vi "Doktorarbeit_Cornelius.vi"(0 "Heizer":refnum<visa-resource-name>="COM1", 1 "Setpoint\n START":bool, 2 "Write to File":bool, 3 "SP 1 shall be (°C)":dbl=20.0 min=0.0 max=999.0, 4 "Intervall (s)":u32=1 max=600, 5 "Write/\nRead":bool=TRUE, 6 "Delay (ms)":u32=500 min=100 max=600000, 7 "Auto Tune":bool, 9 "Standby":bool, 11 "Reset\nSTOPP":bool, 12 "Read Temperature":bool=TRUE, 13 "Get Values":bool, 15 "File Path":path) -> (8 "Temperature (°C)":dbl format="%#.3f", 14 "SP 1 is (°C)":dbl)   [LabVIEW 2010]
doc: "1. Verwendung\n\nDas Programm dient der Steuerung und Abfrage des Thermocontrollers I3252 und dem Auslesen von zwei VC 840 Messgeräten und einem Druckmessgerät Pfeiffer Single Gauge. \nDie Messgeräte werden Standardmäßig ausgelesen und erst nach Betätigung des Schalters \"Write to File\" in einer Textdatei abgespeichert. Das Eingabefeld \"Intervall\" legt den Abstand der Messpunkte fest.\nDer Setpoint für den Thermocontroller wird erst nach Betätigung des Tasters \"Setpoint START\" übernommen und angesteuert. Er wird ind den EEPROM des Gerätes geschrieben. Die Regelung kann mit Hilfe des Schalters \"Standby\" unterbrochen werden. Durch den Taster \"Reset STOPP\" kann der Setpoint aus dem EEPROM gelöscht werden.\nDie Eingabeflächen \"Constant\" und \"Thickness\" dienen der Berechnung des spezifischen Widerstands.\nDie Eingabeflächen \"User\" und \"Sample\" werden in den Header der Textdatei übernommen.\nDer Indikator \"File Path\" zeigt den aktuellen Speicherort der Textdatei an. Dieser wird nach ausschalten des Schalters \"Write to File\" gelöscht. Bei erneuten Schreiben muss ein neuer Speicherort gewählt werden. Bei Wahl desselben Speicherorts werden sämtliche bereits gespeicherte Daten gelöscht.\n\n\n2. Erläuterungen zum Blockdiagramm\n2.1 äußere Sequenz\nDie äußerte Sequenz besteht aus fünf Frames. Der erste dient der Initialisierung der Ports. Der zweite dient als Verzögerung um dem Programm genug Zeit zu geben die Ports zu öffnen. Jedoch senden die beiden VC 840 bereits Informationen an den Computer die in einem Puffer zwischengespeichert werden. Im dritten Frame wird dieser Puffer geleert. Somit kommt es zu keinem Framing Error. Desweiteren wird in diesem Frame die Startzeit der Messungen genommen. Im vierten Frame wird die eigentliche Messung und Verarbeitung der Daten durchgeführt. Die while-Schleife wird nur durch Auftreten eines Fehlers oder durch Betätigung des Stopbuttons auf dem Front Panel in der oberen linken Ecke unterbrochen. Im fünften und letzten Frame werden die Ports wieder geschlossen und beim Auftreten eines Fehlers wird das Programm automatisch gestoppt. Falls kein Fehler auftritt wird die Sequenz von vorne abgearbeitet.\n\n2.2 while-Schleife und innere Sequenz\n2.2.1 \"Event Structure\"\n2.2.1.1 Allgemein\nDer erste Frame beinhaltet ein \"Event Structure\". Dieser reagiert auf insgesamt elf verschiedene Ereignisse. Falls keines dieser Ereignisse auftreten sollte, warte die Struktur eine Millisekunde bevor die \"Event Structure\" verlassen wird. Die übrigen Ereignisse treten ein, wenn der entsprechende Kontroller eine Werteänderung erfährt.\n\n2.2.1.2 Event: Setpoint\nDieser Case besteht von außen nach innen aus einer Stacked Sequence, einer for-Loop und einer Flat Sequence die wiederum zwei \"Case Structures\" enthält. Als erstes wird bei dem Schalter \"Setpoint START\" der Blinkmodus aktiviert und bei dem Schalter \"Read Temperature\" deaktiviert. Danach folgt das eigentliche setzen des Temperatursollwerts. In der ersten Iteration wird dem Controller I3252 ein Schreibbefehl gesendet. Theoretisch kann der Setpoint in den RAM oder in den EEPROM geschrieben werden. Diese Auswahl erfolgt mit Hilfe des Schalters \"RAM\". Da das Schreiben in den RAM -Speicher aber aus diversen Gründen nicht erwünscht ist, wurde es nicht implementiert. Eine nachträgliche Implementierung ist aber leicht möglich, in dem die untere String-Konstante \"*P012\" durch \"*W012\" ersetzt wird. An diesem Befehl wird eine fünfstellige Hexadezimalzahl angehängt, die den Sollwert wiedergibt. Der Sollwert wird vorher mit zehn multipliziert, da das Komma standardmäßig nach der ersten Ziffer festgesetzt wurde (Bsp.: 800 wird gesendet um 80 einzustellen). Dieser Befehlsstrang wird an das Gerät mittels des SubVIs \"Comm_Interface\", auf welches später noch näher eingegangen wird, weitergegeben. Der durch das Gerät zurückgegebene String wird nicht verarbeitet.\nDie zweite Iteration dient dem Auslesen des eingestellten Sollwertes. Wahlweise kann der RAM- oder der EEPROM-Speicher ausgelesen werden. Die eigentliche Verarbeitung des Ausgabestrings erfolgt durch das SubVI \"Edit Setpoint\".\nDie Implementierung zur Einstellung des zweiten Setpoints erfolgt durch kopieren der ersten beiden Fälle und ersetzen der \"1\" im Befehf durch eine \"2\" (Bsp.: \"*P012\" zu \"*P022\"). Es darf aber nicht vergessen werden, dass dann ebenfalls die Anzahl der Iterationen angepasst werden muss.\nAls letztes wird der Blinkmodus des Schalters \"Setpoint START\" wieder deaktiviert.\n\n2.2.1.3 Event: Standby\nDieses Ereignis aktiviert bzw. deaktiviert als erstes den Blinckmodus des entsprechenden Schalters und sendet danach den Befehl zum aktivieren (\"*D03\") oder zum deaktivieren (\"*E03\") des Standbymodus an den Thermocontroller.\n\n2.2.1.4 Event: Set Command \nDer in das Feld \"Command shall be\" eingegebene Befehl wird an den Thermocontroller übermittlet. Die korrekte Form des Befehls ist im \"Communication Manuel\" nachzuschlagen. Das \"*\"-Zeichen wurde allerdings schon implementiert und muss somit nicht mit eingegeben werden.\n\n2.2.1.5 Event: Reset\nIn der ersten Iteration wird der Reset-Befehl an den Thermocontroller gesendet. In Folge wird der gesamte EEPROM-Speicher gelöscht. Deshalb wird in der zweiten Iteration der Setpoint aktualisiert. Dieser Befehl hat keinen Einfluss auf den RAM-Speicher. Die anschließende Wartezeit ist auf vier Sekunden festgesetzt und wurde empirisch ermittelt. Diese Zeit benötigt das Gerät um den Reset durchzuführen und für die Kommunikation wieder zur Verfügung zu stehen.\n\n2.2.1.6 Event: Auto Tune\nEs ist festgeschrieben, dass der Setpoint für die \"Auto Tune\"-Funktion wenigstens 20°C über der aktuellen Temperatur liegt. Deshalb wird zunächst der aktuelle Temperaturwert ausgelesen. Im zweiten Schritt werden zu diesem Wert zwanzig addiert und der Setpoint wird in den RAM-Speicher geschrieben. Das Schreiben in diesen Speicher ist nötig, da die \"Auto Tune\"-Funktion\" erst nach einem Reset startet. Im dritten Schritt wird der eigentliche Befehl für den \"Auto Tune\" gesendet (siehe dazu \"Communication Manuel\" S.27). Als vierte und letzte Iteration der for-Schleife folgt der bereits erwähnte Reset-Befehl. Der Temperatursollwert, der im RAM-Speicher eingetragen ist, muss zum Schluss wieder auf 0°C gesetzt werden. Die Zeit für die Ausführung des \"Auto Tune\"-Befehls wurde empirisch ermittelt und 45 s festgesetzt.\n\n2.2.1.7 Event: Write LOW/HI\nDieses Ereignis setzt die am Analogausgang anliegende Spannung fest. Normalerweise beträgt dieser Spannungswert 0-10 V. Das angeschlossene Netzteil verträgt aber maximal nur 2,3 V. Aus diesem Grund wird der \"%HIGH\" auf 23 gesetzt. Somit beträgt die maximal anliegende Spannung nur noch 23% von der maximal möglichen, d.h 2,3V. Ein niedrigerer Wert ist jederzeit möglich, genauso wie ein höherer für den Parameter \"%LOW\". Diese werden zunächst nacheinander in den RAM-Speicher geschrieben und anschließend wieder ausgelesen.\n\n2.2.1.8 Event: Set PID\nDie Werte für den PID-Regler können sowohl mit Hilfe der \"Auto Tune\"-Funktion, als auch manuell eingestellt werden. Es wird wiederum zwischen dem Schreiben in den RAM- und dem EEPROM-Speicher unterschieden. Zunächst werden die Werte für \"P\", \"I\" und \"D\", in dieser Reihenfolge, gesetzt und danach die aktuellen Werte ausgelesen.\n\n2.2.1.9 Event: Get Values\nDieses Ereignis hat zur Folge, dass die Werte für \"P\", \"I\", \"D\", \"%LOW\", \"%HIGH\" und des Setpoints wahlweise aus dem RAM- oder EEPROM-Speicher gelesen werden. Die aktuellen Werte werden nicht nur in die entsprechenden Anzeigefelder übernommen, sondern auch in die entsprechenden Eingabefelder, mit Ausnahme des Temperatursollwerts. \n\n2.2.1.10 Event: RAM\nPrinzipiell kann zwischen dem Schreiben in den RAM- oder EEPROM-Speicher des Thermocontrollers gewählt werden. Die entsprechende Schalterposition auf dem Frontpanel zeigt den aktuell verwendeten Speicher an. Die Anzeigewerte werden bei jedem Umschalten aktualisiert und sind im entsprechenden Speicher eingetragen. Die Implementierung ist identisch mit der des Ereignisses \"Get Values\". Es gilt zu beachten, dass die Werte für \"%LOW\" und \"%HIGH\" nur in den RAM-Speicher geschrieben werden können und somit auch nur aus diesem ausgelesen werden können.\n\n2.2.1.11 Event: Set Gauge to Zero\nMit Hilfe der SubVIs \"Get Pressure\" und \"Offset Display\" werden die Werte für den alten und den neuen Offset und der durch den zweiten Drucksensor ermittelt Druck ermittelt. \n\n2.2.1.12 Event: Write to File\nSollte der Schalter \"Write to File\" aktiviert werden, d.h. Schalterposition oben, so wird zunächst durch das SubVI \"Header\" ein Header für die unter \"File Path\" definierte Datei angelegt. Alle Werte, die bereits in der entsprechenden Datei stehen, werden dabei gelöscht.\n\n2.2.2 \"Timed Structures\"\nIm dritten Frame der inneren Sequenz werden die Werte für Zeitpunkt, Temperatur, Spannung, Strom und Druck ermittelt. Damit die Werte zum gleichen Zeitpunkt aufgenommen werden, werden \"Timed Sequences\" eingesetzt. Mit dem entsprechenden Schalter auf dem Front Panel unter dem Tab \"Settings\" kann gewählt werden, ob das entsprechende Gerät ausgelesen werden soll oder nicht. Die einzelnen Sequenzen werden parallel abgearbeitet, womit die Prozesszeit von diesem Frame durch der zeitintensivsten Sequenz abhängt. Dies ist in aller Regel das Auslesen der Temperatur, da ein \"Delay\" von 500 ms oder größer benötigt wird, um den Controller ordentlich ansprechen zu können.\nDie Systemzeit wird durch das SubVI \"System Time in Seconds\" in Sekunden umgerechnet und der in dem Parameter \"Starttime\" gespeicherte Wert wird abgezogen. Somit werden die Sekunden seit dem Start des Programms gezählt.\n\n2.2.3 restlichen Frames\nIm zweiten Frame wird das Intervall zwischen den einzelnen Messwerten festgelegt. Dabei wird der Wert des Parameters \"Delay\" abgezogen. Dieser Wert beträgt im Normalfall 500 ms und ist somit nicht vernachlääsigbar.\nDer Vierte Frame beinhaltet die Umrechnung des Temperatur-Strings in einen Temperaturwert durch das SubVI \"Edit Tmperature\", die Berechnung des spezifischen Widerstands durch das SubVI \"Resistivity Calculation\" und die Überprüfung des Druckwerts. Auch werden die neu gewonnen Werte in das entsprechende Shift-Register übernommen. Falls der Druckwert einen in dem Parameter \"Pressure Limit (mbar)\" festgelegten Grenzwert überschreiten sollte, wird der Thermocontroller automatisch in den Standby-Modus versetzt. Des Weiteren wird der Schalter \"Standby\" solange gesperrt, wie der Druck oberhalb des Grenzwertes liegt. Wenn der Druck wieder unter den Grenzwert gesunken ist, wird der Standby-Befehl nicht automatisch aufgehoben, sondern muss vom Benutzer durch Betätigung des entsprechenden Schalters gegeben werden.\nIm fünften Frame werden die Diagramme erstellt. Dabei wird jedes Mal von neuem das gesamte Shift-Register als Graph dargestellt. Weiterhin werden die Messwerte in ein 1D-Array geschrieben.\nDer sechste und letzte Frame beinhaltet den eigentlich Schreibvorgang der Messwerte in eine Textdatei und die Überprüfung ob ein Fehler vorliegt.\n\n2.3 SubVIs\n2.3.1 Allgemein\nDie SubVIs für die Messgeräte VC840 und das Druckmessgerät wurden aus anderen Quellen übernommen. \n\n2.3.2 \"Header\"\nIn den Header wird zunächst das aktuelle Datum und die aktuelle Zeit übernommen. Die ausgewählte Datei wird dabei überschrieben. Danach wird der Name des Benutzers und der Probe übernommen. Zum Schluss werden die Einheiten in einer Reihe, durch einen Tabulator getrennt, in den Header geschrieben.\n\n2.3.3 \"I3252 Comm Interface\"\nDieses VI stellt die Kommunikation mit dem Thermocontroller her und gibt den Ausgabe-String zurück.\n\n2.3.4 \"I3252 Edit Setpoint\"\nIm Ausgabe-String vom Thermocontroller ist an der vierten Stelle die Stelle des Dezimalpunktes verschlüsselt. Dieses Hexadezimalzahl wird herausgefiltert und an ein \"ENUM Controller\" übergeben. Dieser weist der Hexadezimalzahl eine Nummer zu, mit welcher ein Wert aus einem Array entnommen wird. Dieser Wert dient als Quotient. Der tatsächliche Wert kann somit errechnet werden.\n\n2.3.5 \"I3252 Edit Temperature\"\nDer Temperatur-String, der vom Thermocontroller zurückgegeben wird, wird in eine Dezimalzahl umgewandelt. Manchmal kommt es aus zu Dropouts, die durch dieses Programm herausgefiltert werden. Der letzte Wert wird dabei in einer \"Feedback Node\" gehalten unter der Annahme, dass sich der Temperaturwert nicht sprunghaft ändert.\n\n2.3.6 \"Resistivity Calculation\"\nDer spezifische Widerstand wird nach folgender Formel ausgerechnet. Dabei entspricht t der Dicke der Probe und C ist eine Konstante.\nrho=C*pi*t*U/(ln( 2)*I)\n\n2.3.7 \"System Time in Seconds\"\nZunächst wird die aktuelle Systemzeit ausgelesen. Danach wird diese in Stunden, Minuten und Sekunden aufgeteilt, alles in Sekunden umgerechnet und letztendlich addiert."
uses:
  <vilib>/Platform/TimedLoop/XDataNode/XDataNode.xnode
  <vilib>/Platform/TimedLoop/XDataNode/timing_clust.ctl
  <vilib>/Platform/TimedLoop/XDataNode/nitl_modes.ctl
  <vilib>/Platform/TimedLoop/XDataNode/wakeup.ctl
  <vilib>/Instr/_visa.llb/VISA Configure Serial Port (Instr).vi
  <vilib>/Platform/TimedLoop/scheduler/LVUserAPI/_suppVIs/Create_1kHz_TSource.vi
  <vilib>/Utility/file.llb/Write To Spreadsheet File (DBL).vi
  <vilib>/Platform/TimedLoop/XDataNode/XDNodeRunTimeDep.lvlib
panel:
  out "appended array":dbl[](array[numeric])
  in  "Tab Control":T1(tab)
  out "Pressure":cluster{dbl[], dbl[]}(graph)
  out "Pressure (mbar)":dbl format="%.2e"
  in  "Thickness (nm)":dbl min=0.0
  in  "Constant":dbl=4.532 min=0.0 max=5.0
  in  "Sample":string
  in  "User":string
  out "Temperature":cluster{dbl[], dbl[]}(graph)
  out "Resistivity":cluster{dbl[], dbl[]}(graph)
  out "Resistivity (Ohm*cm)":dbl format="%.3e"
  out "current time (s)":dbl
  out "data logger intervall (s)":dbl
  out "loop time (s)":dbl
  in  "Pressure Limit (mbar)":dbl=0.0001 min=0.0 max=1100.0
  out "Pressure 1 (mbar)":dbl
  out "Current Offset (mbar)":dbl
  out "Old Offset (mbar)":dbl
  out "Pressure 2 (mbar)":dbl
  out "Status":T2(ring)
  in  "Sensor Nr.:":enum16{"sensor 1", "aensor 2", "test"}(ring)
  in  "Port":T3(ring)=enum."COM 5"
  in  "Set Gauge to Zero":bool
  out "Error Out":bool
  in  "VC 840 2":refnum<visa-resource-name>="COM4"
  out "Reading 2":dbl format="%_4f"
  out "Mode 2":enum16{"?", "Diode", "Beep", "DC", "AC"}(ring)
  out "Unit 2":string
  in  "VC 840 1":refnum<visa-resource-name>="COM3"
  out "Reading 1":dbl format="%_4f"
  out "Mode 1":enum16{"?", "Diode", "Beep", "DC", "AC"}(ring)
  out "Unit 1":string
  out "Status 1":T4
  out "Status 2":T4
  in  "Set Command":bool
  in  "Set PID":bool
  in  "Write LOW/HI":bool
  out "% HIGH is":u32
  out "% LOW is":u32
  in  "% High shall be":u32=23 max=24
  in  "% LOW shall be":u32 max=25
  in  "Flow Control":u16(ring) items=["None"=0, "XON/XOFF"=1, "RTS/CTS"=2, "DTR/DSR"=4]
  in  "Stop Bits":u16(ring)=10 items=["1.0"=10, "1.5"=15, "2.0"=20]
  in  "Parity":u16(ring)=1 items=["None", "Odd", "Even", "Mark", "Space"]
  in  "Data Bits":u16=7 min=5 max=8 step=1
  in  "Baud Rate":u32=9600
  out "Command is":string
  in  "Command shall be":string
  in  "RAM":bool=TRUE caption="EEPROM"
  out "D (Rate) is":u32
  out "I ( Reset1) is":u32
  out "P (PB1) is":u32
  in  "D (Rate) shall be":u32 max=3999
  in  "I ( Reset1) shall be":u32 max=3999
  in  "P (PB1) shall be":u32 max=9999
  in  "Read VC 840 1":bool=TRUE
  in  "Read VC 840 2":bool=TRUE
  in  "Read Pressure":bool=TRUE
  out "Current":cluster{dbl[], dbl[]}(graph)
  out "Voltage":cluster{dbl[], dbl[]}(graph)
  out "Voltage (V)":dbl format="%.4e"
  out "Current (A)":dbl format="%.4e"
  # "I3252 Control"
  # "VC 840 Control"
  # "Pfeiffer Control"
  # "Authors:  Daniel Schuster (sir-dan@web.de)\n                 Steffen Cornelius (s.cornelius@hzdr.de)\n\n                 premade SubVIs for readout of Pfeiffer gauge and VC840 Multimeters were used\n                 SubVI \"I3252_Comm_Interface\" is based on a modified Labview example\n\nRelease:  v1.0    \n\nVersion History:\n\nv1.1  28.06.2011\n             - Format des Files geändert von %.3f auf %g\n             - maximale Eingabewerte für PID begrenzt\nv1.2  12.07.2011\n             - Anzeige p,rho, U, V auf Scientific geändert\n             - y-Achse p,rho auf Log geändert\n             - numerische Zeitanzeige hinzugefügt\n             - 4PP Constant: pi/ln(2)=4,532 set as the default value\nv1.3  25.07.2011\n             - Zeitvariable auf EXT geändert, um Sprünge in Diagrammen loszuwerden\nv1.4 27.07.2011\n             - ALLE Variablen auf DBL zurückgesetzt wegen Formatierungsproblem im File\n             - Zeitberechnung neu gemacht (Tick count differenzen) -> Zeitsprünge korrigiert ?\n             - Delay/Intervall überarbeitet"
  # "Version 1.4    - last change 27.07.2011"
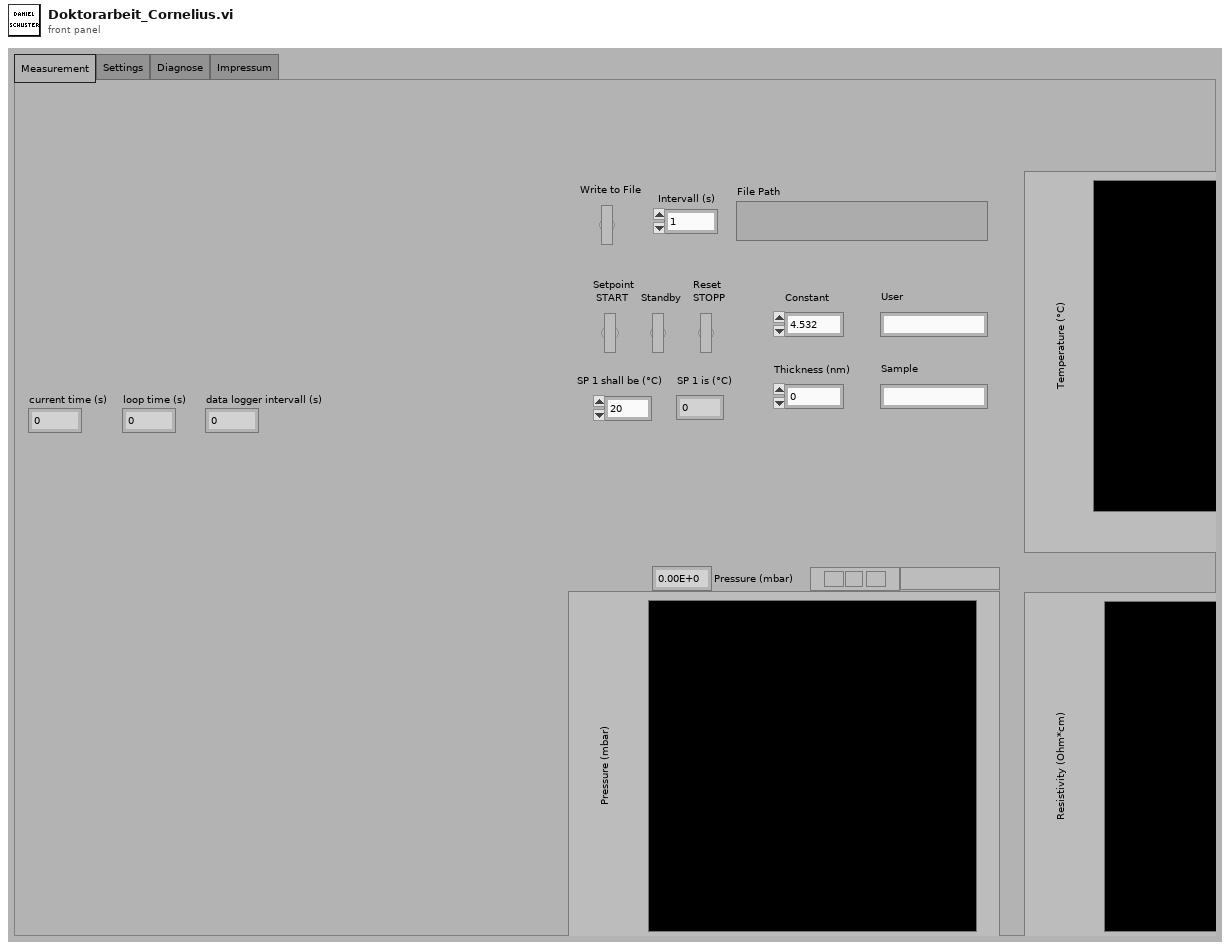
[diagram p1: front panel]
types:
  T1 = enum32{"Measurement", "Settings", "Diagnose", "Impressum"}
  T2 = enum16{"data OK", "underrange", "overrange", "sensor error", "sensor off", "no sensor", "ID error"}
  T3 = enum16{"COM 1", "COM 2", "COM 3", "COM 4", "COM 5", "COM 6", "COM 7", "COM 8", "COM 9", "COM 10", "COM 11", "COM 12"}
  T4 = cluster{"Low Bat":bool, "Auto":bool, "Delta":bool, "Hold":bool, "RS232":bool}
  T5 = typedef "XDNodeRunTimeDep.lvlib/timing_clust.ctl" = cluster{"Expected End [f-1]":u64, "Actual End [f-1]":u64, "Finished Late? [f-1]":bool, "Expected End [i-1]":u64, "Actual End [i-1]":u64, "Finished Late? [i-1]":bool, "Expected Start [i]":u64, "Actual Start [i]":u64, "Expected Start [f]":u64, "Actual Start [f]":u64, "Source Name":string, "Structure Name":string, "Period":i64, "Deadline":i64, "Offset":i64, "Start":i64, "Priority":i32, "Timeout":i32, "Mode":T6, "Wakeup Reason":T7, "Error":errorcluster, "Source Type":string, "Secondary Source Type":string, "Global End Time":u64, "Global Start Time":u64, "Frame Duration":u64, "Iteration Duration":u64, "Assigned CPU":i32, "I/O Scan Engine Mode":u32}
  T6 = typedef "XDNodeRunTimeDep.lvlib/nitl_modes.ctl" = enum32{"No Change", "Process missed periods, maintain original phase", "Discard missed periods, maintain original phase", "Process missed periods, ignore original phase", "Discard missed periods, ignore original phase"}
  T7 = typedef "XDNodeRunTimeDep.lvlib/wakeup.ctl" = enum32{"Normal", "Aborted", "Asynchronous wakeup", "Timing source error", "Timed loop error", "Timeout"}
  T8 = enum8{"Enabled", "Disabled", "Disabled and Grayed Out"}
  T9 = cluster{"VISA resource name out":refnum<visa-resource-name>, "error out":errorcluster, "Delay (ms)":u32, "Write/\nRead":bool}
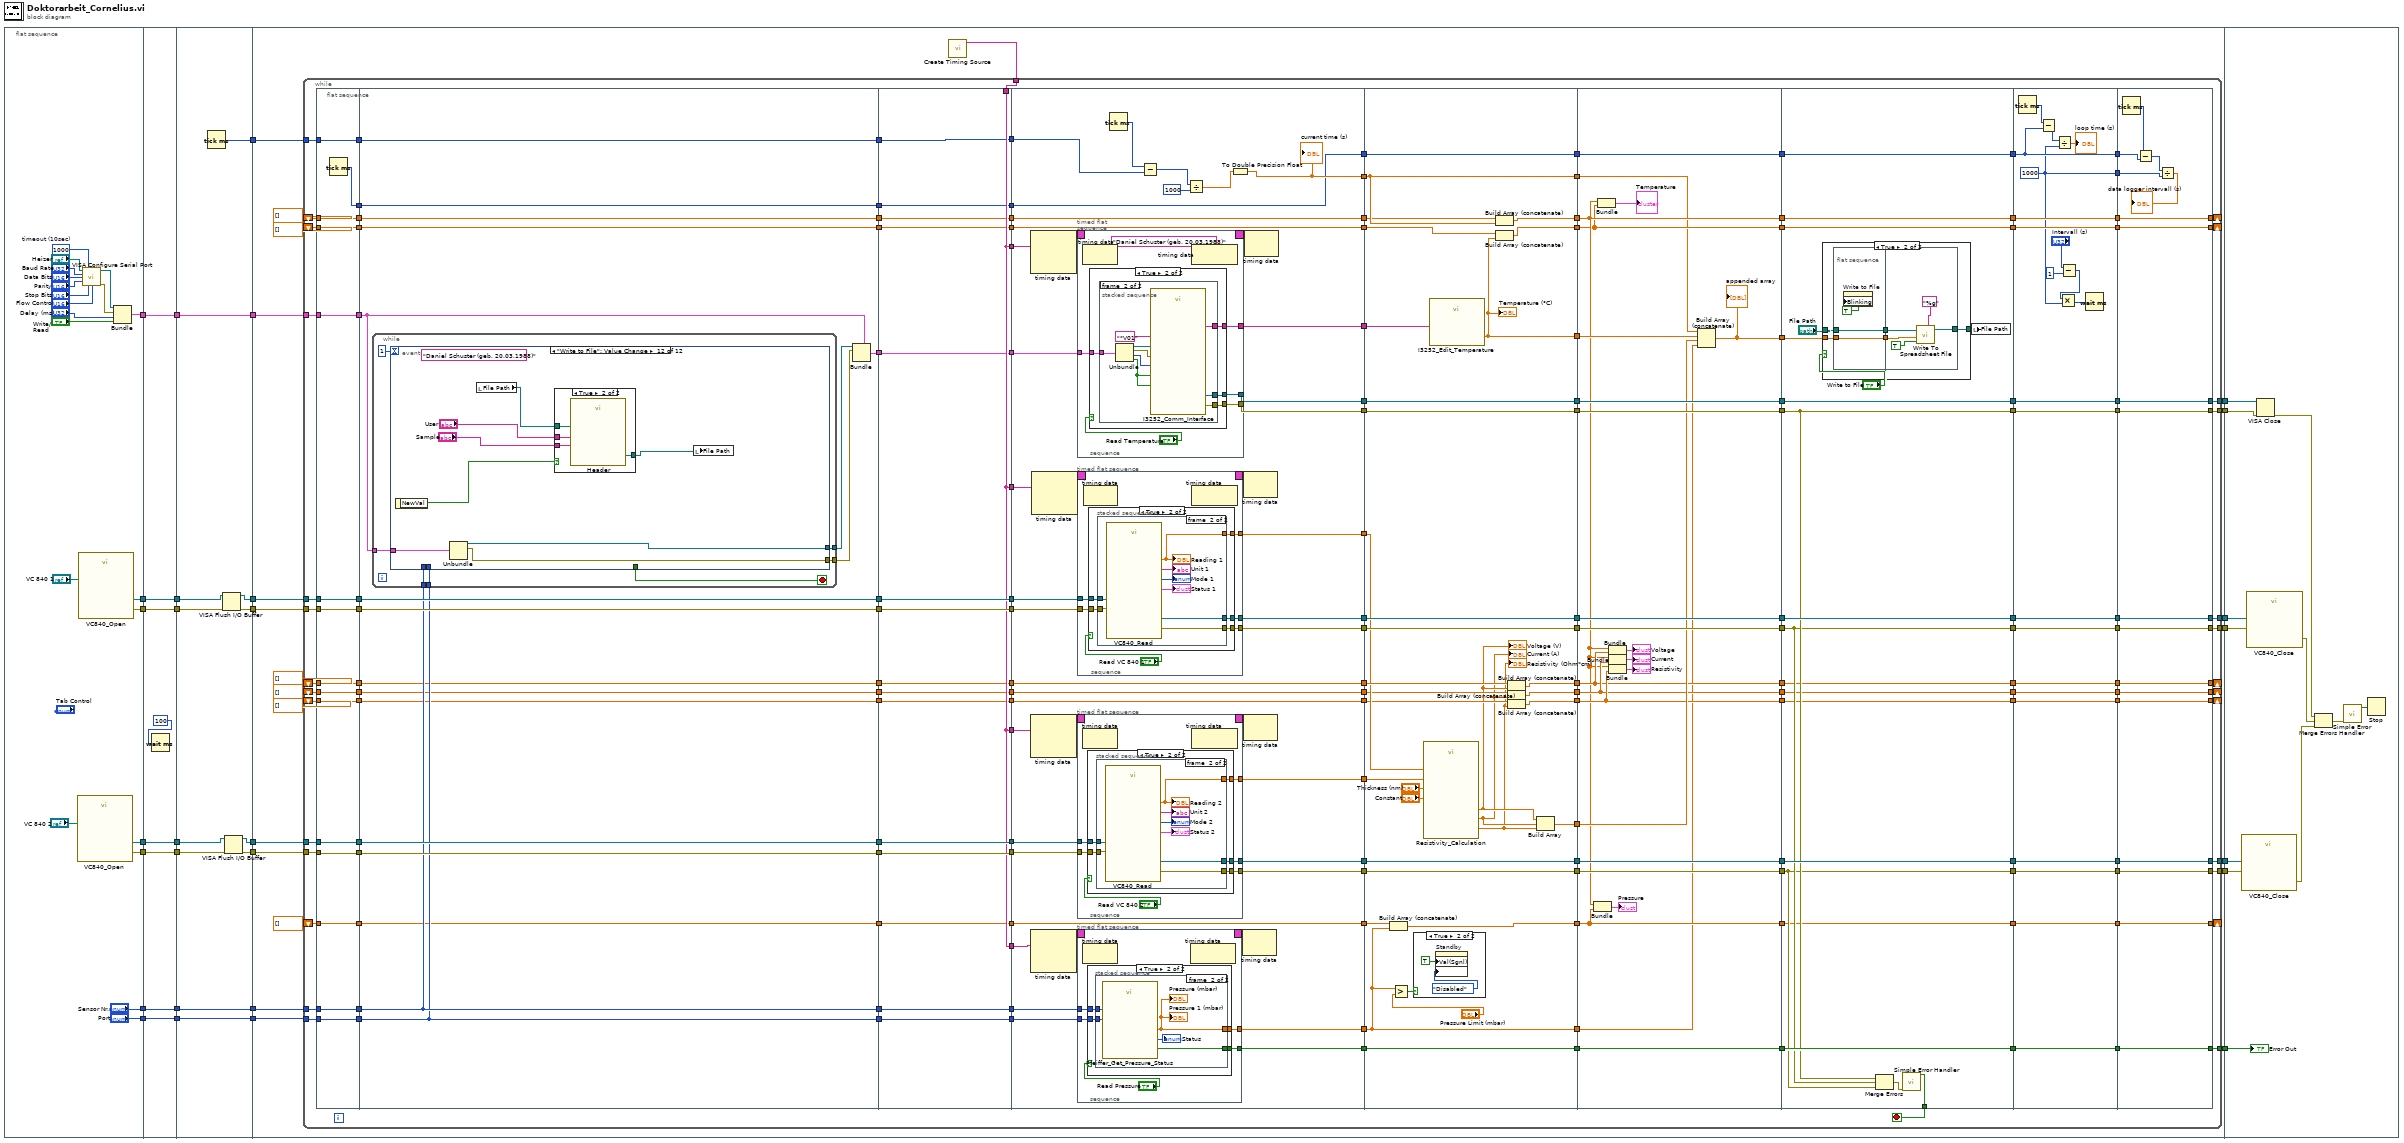
[diagram p0: block diagram]
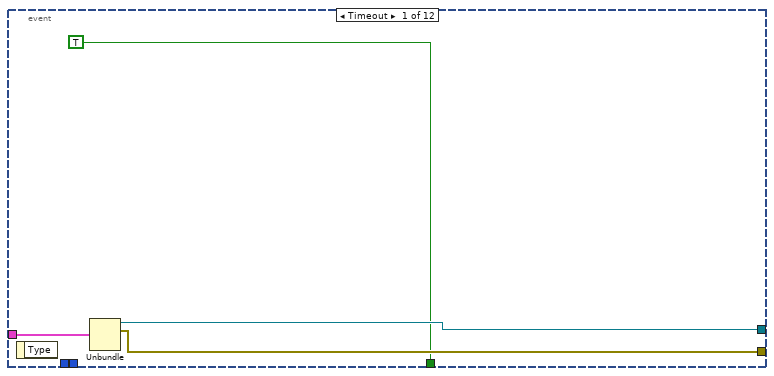
[diagram p2: hidden frame]
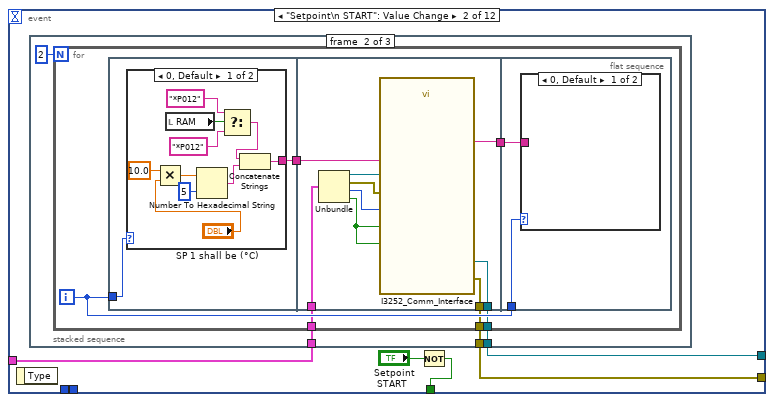
[diagram p3: hidden frame]
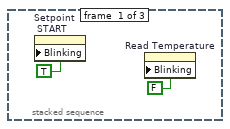
[diagram p4: hidden frame]
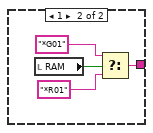
[diagram p5: hidden frame]
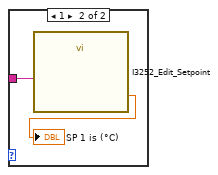
[diagram p6: hidden frame]
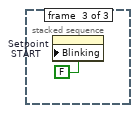
[diagram p7: hidden frame]
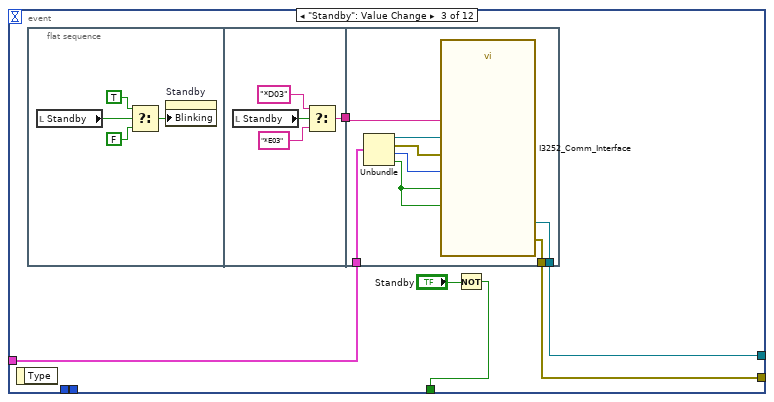
[diagram p8: hidden frame]
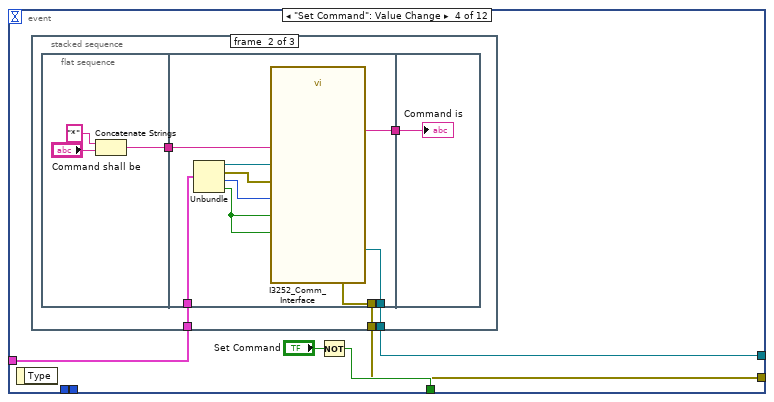
[diagram p9: hidden frame]
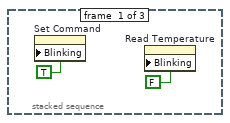
[diagram p10: hidden frame]
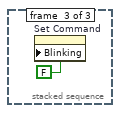
[diagram p11: hidden frame]
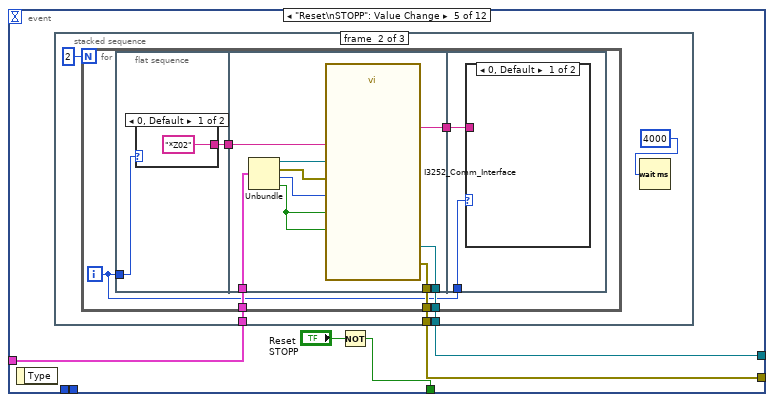
[diagram p12: hidden frame]
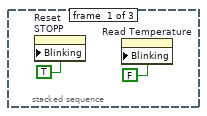
[diagram p13: hidden frame]
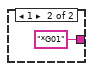
[diagram p14: hidden frame]
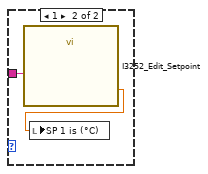
[diagram p15: hidden frame]
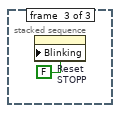
[diagram p16: hidden frame]
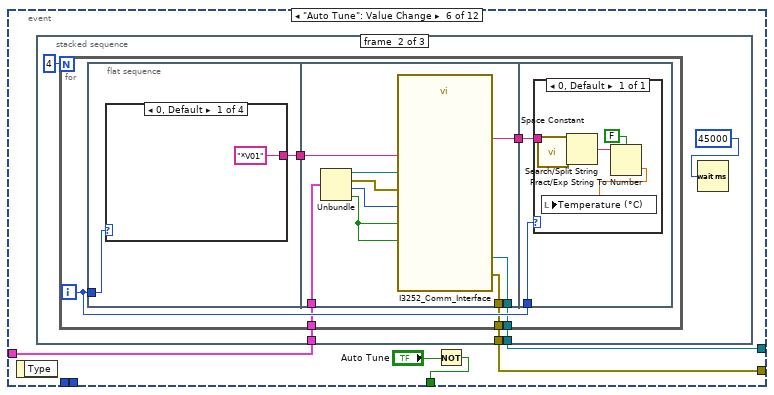
[diagram p17: hidden frame]
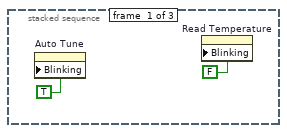
[diagram p18: hidden frame]
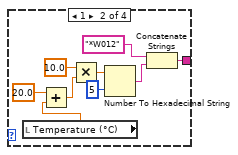
[diagram p19: hidden frame]
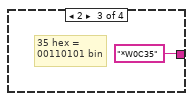
[diagram p20: hidden frame]
diagram:
  n1 = flat-sequence {
    tunnel: [w48] -> w22
    tunnel: [w49] -> w21
    tunnel: [w32] -> w20
    tunnel: [w47] -> w19
    tunnel: [w46] -> w18
    tunnel: ["Port"] -> w17
    tunnel: ["Sensor Nr.:"] -> w16
    tunnel: w22 -> [w57]
    tunnel: [w57] -> w15
    tunnel: w21 -> [w56]
    tunnel: [w56] -> w13
    tunnel: w20 -> [w55]
    tunnel: [w55] -> w11
    tunnel: w19 -> [w54]
    tunnel: [w54] -> w9
    tunnel: w18 -> [w53]
    tunnel: [w53] -> w7
    tunnel: w17 -> [w52]
    tunnel: [w52] -> w5
    tunnel: w16 -> [w51]
    tunnel: [w51] -> w3
    tunnel: w15 -> [w61]
    tunnel: [w60] -> w14
    tunnel: w13 -> [w62]
    tunnel: [w59] -> w12
    tunnel: w11 -> [w69]
    tunnel: [w69] -> w10
    tunnel: w9 -> [w64]
    tunnel: [w65] -> w8
    tunnel: w7 -> [w63]
    tunnel: [w66] -> w6
    tunnel: w5 -> [w68]
    tunnel: [w68] -> w4
    tunnel: w3 -> [w67]
    tunnel: [w67] -> w2
    tunnel: [w58] -> w1
    tunnel: w14 -> [w91]
    tunnel: w12 -> [w90]
    tunnel: w10 -> [w89]
    tunnel: w8 -> [w87]
    tunnel: w6 -> [w86]
    tunnel: w4 -> [w79]
    tunnel: w2 -> [w78]
    tunnel: [w85] -> w29
    tunnel: [w84] -> w28
    tunnel: [w83] -> w27
    tunnel: [w82] -> w26
    tunnel: [w81] -> w25
    tunnel: [w80] -> w24
    tunnel: [w77] -> w23
    tunnel: w1 -> [w70]
    tunnel: w29 -> [w1122]
    tunnel: w28 -> [w1121]
    tunnel: w27 -> [w1124]
    tunnel: w26 -> [w1123]
    tunnel: w25 -> [w1126]
    tunnel: w24 -> [w1125]
    tunnel: w23 -> [w1120]
    frame #0 {
      w33 = u32 1000  # timeout (10sec)
      n2 = call "VC840_Open.vi"("VISA resource name"="VC 840 2") -> ("error out"=w46:errorcluster, "VISA resource name out"=w47:refnum<visa-resource-name>)  [unwired: 1 in, 8 out]
      n3 = call "VC840_Open.vi"("VISA resource name"="VC 840 1") -> ("error out"=w49:errorcluster, "VISA resource name out"=w48:refnum<visa-resource-name>)  [unwired: 1 in, 8 out]
      n4 = call-poly "VISA Configure Serial Port"("VISA resource name"="Heizer", "timeout (10sec)"=w33, "baud rate (9600)"="Baud Rate", "data bits (8)"="Data Bits", "parity (0:none)"="Parity", "stop bits (10: 1 bit)"="Stop Bits", "flow control (0:none)"="Flow Control") -> ("VISA resource name out"=w42:refnum<visa-resource-name>, "error out"=w43:errorcluster)  [unwired: 2 in, 5 out]
      n5 = Bundle("VISA resource name out"=w42, "error out"=w43, "Delay (ms)"="Delay (ms)", "Write/\nRead"="Write/\nRead") -> (w32:T9)  [unwired: 1 in]
    }
    frame #1 {
      n6 = Wait (ms)(milliseconds to wait=u32 100) -> ()  [unwired: 1 out]
    }
    frame #2 {
      n7 = Tick Count (ms)() -> (millisecond timer value=w58:u32)
      n8 = VISA Flush I/O Buffer(VISA resource name=w61, error in (no error)=w62) -> (VISA resource name out=w60:refnum<visa-resource-name>, error out=w59:errorcluster)  [unwired: 1 in]
      n9 = VISA Flush I/O Buffer(VISA resource name=w64, error in (no error)=w63) -> (VISA resource name out=w65:refnum<visa-resource-name>, error out=w66:errorcluster)  [unwired: 1 in]
    }
    frame #3 {
      n10 = call-poly <vilib>:"Create Timing Source.vi"() -> ("name (out)"=w88:string)  [unwired: 10 in, 1 out]
      n11 = while {
        tunnel: w91 -> [w250]
        tunnel: w90 -> [w249]
        tunnel: w89 -> [w248]
        tunnel: w88 -> [w241]
        tunnel: w87 -> [w234]
        tunnel: w86 -> [w233]
        tunnel: [w229] -> w85
        tunnel: [w228] -> w84
        tunnel: [w226] -> w83
        tunnel: [w224] -> w82
        tunnel: [w222] -> w81
        tunnel: [w220] -> w80
        tunnel: w78 -> [w216]
        tunnel: w79 -> [w214]
        tunnel: [w212] -> w77
        shift-right: [w178] -> _
        shift-left: dbl[] [] -> [w183]
        shift-right: [w154] -> _
        shift-left: dbl[] [] -> [w197]
        shift-right: [w180] -> _
        shift-left: dbl[] [] -> [w187]
        shift-right: [w151] -> _
        shift-left: dbl[] [] -> [w196]
        shift-right: [w190] -> _
        shift-left: dbl[] [] -> [w193]
        shift-right: [w148] -> _
        shift-left: dbl[] [] -> [w195]
        tunnel: w70 -> [w141]
        stop <- w144 stop-if-true
        n12 = flat-sequence {
          tunnel: w141 -> [w252]
          tunnel: w183 -> [w253]
          tunnel: w187 -> [w254]
          tunnel: w193 -> [w255]
          tunnel: w195 -> [w256]
          tunnel: w196 -> [w257]
          tunnel: w197 -> [w258]
          tunnel: w214 -> [w259]
          tunnel: w216 -> [w260]
          tunnel: w233 -> [w261]
          tunnel: w234 -> [w262]
          tunnel: w248 -> [w263]
          tunnel: w249 -> [w264]
          tunnel: w250 -> [w265]
          tunnel: [w265] -> w140
          tunnel: [w264] -> w139
          tunnel: [w263] -> w138
          tunnel: [w262] -> w137
          tunnel: [w261] -> w136
          tunnel: [w260] -> w135
          tunnel: [w259] -> w134
          tunnel: [w258] -> w133
          tunnel: [w257] -> w132
          tunnel: [w256] -> w131
          tunnel: [w255] -> w130
          tunnel: [w254] -> w129
          tunnel: [w253] -> w128
          tunnel: [w252] -> w127
          tunnel: [w251] -> w107
          tunnel: [w283] -> w247
          tunnel: [w282] -> w245
          tunnel: [w278] -> w243
          tunnel: [w277] -> w238
          tunnel: [w276] -> w236
          tunnel: [w275] -> w215
          tunnel: [w274] -> w213
          tunnel: [w273] -> w194
          tunnel: [w272] -> w188
          tunnel: [w271] -> w184
          tunnel: [w270] -> w162
          tunnel: [w269] -> w159
          tunnel: [w268] -> w157
          tunnel: [w267] -> w142
          tunnel: w140 -> [w283]
          tunnel: w139 -> [w282]
          tunnel: w138 -> [w281]
          tunnel: w137 -> [w277]
          tunnel: w136 -> [w276]
          tunnel: w135 -> [w275]
          tunnel: w134 -> [w274]
          tunnel: w133 -> [w270]
          tunnel: w132 -> [w269]
          tunnel: w131 -> [w268]
          tunnel: w130 -> [w273]
          tunnel: w129 -> [w272]
          tunnel: w128 -> [w271]
          tunnel: w127 -> [w267]
          tunnel: [w266] -> w108
          tunnel: w107 -> [w266]
          tunnel: w247 -> [w810]
          tunnel: [w810] -> w246
          tunnel: w245 -> [w809]
          tunnel: [w809] -> w244
          tunnel: w243 -> [w803]
          tunnel: [w803] -> w242
          tunnel: w241 -> [w804]
          tunnel: [w804] -> w240
          tunnel: [w804] -> w239
          tunnel: w238 -> [w808]
          tunnel: [w808] -> w237
          tunnel: w236 -> [w807]
          tunnel: [w807] -> w235
          tunnel: [w804] -> w232
          tunnel: [w806] -> w218
          tunnel: [w805] -> w217
          tunnel: w215 -> [w806]
          tunnel: w213 -> [w805]
          tunnel: [w804] -> w210
          tunnel: w194 -> [w802]
          tunnel: [w802] -> w191
          tunnel: w188 -> [w801]
          tunnel: [w801] -> w186
          tunnel: w184 -> [w800]
          tunnel: [w800] -> w181
          tunnel: [w799] -> w163
          tunnel: w162 -> [w799]
          tunnel: [w798] -> w160
          tunnel: w159 -> [w798]
          tunnel: [w797] -> w158
          tunnel: w157 -> [w797]
          tunnel: [w796] -> w143
          tunnel: w142 -> [w796]
          tunnel: [w795] -> w109
          tunnel: w108 -> [w795]
          tunnel: [w817] -> w209
          tunnel: w246 -> [w851]
          tunnel: w244 -> [w850]
          tunnel: w242 -> [w847]
          tunnel: w240 -> [w846]
          tunnel: w239 -> [w845]
          tunnel: w237 -> [w832]
          tunnel: w235 -> [w831]
          tunnel: w232 -> [w833]
          tunnel: [w829] -> w208
          tunnel: [w830] -> w207
          tunnel: [w844] -> w206
          tunnel: [w843] -> w205
          tunnel: [w842] -> w204
          tunnel: [w841] -> w203
          tunnel: w218 -> [w840]
          tunnel: w217 -> [w839]
          tunnel: [w836] -> w202
          tunnel: w210 -> [w828]
          tunnel: [w827] -> w201
          tunnel: [w826] -> w200
          tunnel: [w825] -> w199
          tunnel: [w824] -> w198
          tunnel: [w823] -> w192
          tunnel: w191 -> [w823]
          tunnel: w186 -> [w822]
          tunnel: [w822] -> w185
          tunnel: [w821] -> w182
          tunnel: w181 -> [w821]
          tunnel: w163 -> [w820]
          tunnel: [w820] -> w161
          tunnel: w160 -> [w819]
          tunnel: w158 -> [w818]
          tunnel: [w819] -> w156
          tunnel: [w818] -> w155
          tunnel: w143 -> [w816]
          tunnel: [w812] -> w110
          tunnel: w109 -> [w812]
          tunnel: w209 -> [w1001]
          tunnel: [w998] -> w176
          tunnel: w208 -> [w1017]
          tunnel: [w1017] -> w175
          tunnel: w207 -> [w1016]
          tunnel: [w1016] -> w174
          tunnel: w206 -> [w1015]
          tunnel: [w1015] -> w173
          tunnel: w205 -> [w1014]
          tunnel: [w1014] -> w172
          tunnel: w204 -> [w1013]
          tunnel: [w1013] -> w171
          tunnel: w203 -> [w1012]
          tunnel: [w1012] -> w170
          tunnel: [w1003] -> w169
          tunnel: w202 -> [w1011]
          tunnel: [w1011] -> w168
          tunnel: w201 -> [w995]
          tunnel: w200 -> [w1005]
          tunnel: w199 -> [w1003]
          tunnel: w198 -> [w1006]
          tunnel: [w1001] -> w167
          tunnel: w192 -> [w1004]
          tunnel: [w1002] -> w166
          tunnel: w185 -> [w1000]
          tunnel: w182 -> [w999]
          tunnel: [w997] -> w165
          tunnel: [w985] -> w164
          tunnel: w161 -> [w996]
          tunnel: w156 -> [w993]
          tunnel: w155 -> [w992]
          tunnel: [w994] -> w152
          tunnel: [w991] -> w149
          tunnel: [w990] -> w146
          tunnel: [w986] -> w145
          tunnel: [w984] -> w111
          tunnel: w110 -> [w984]
          tunnel: w176 -> [w1036]
          tunnel: [w1044] -> w231
          tunnel: [w1043] -> w230
          tunnel: w175 -> [w1043]
          tunnel: [w1037] -> w227
          tunnel: w174 -> [w1037]
          tunnel: [w1042] -> w225
          tunnel: w173 -> [w1042]
          tunnel: [w1041] -> w223
          tunnel: w172 -> [w1041]
          tunnel: [w1040] -> w221
          tunnel: w171 -> [w1040]
          tunnel: [w1039] -> w219
          tunnel: w170 -> [w1039]
          tunnel: w169 -> [w1022]
          tunnel: [w1038] -> w211
          tunnel: w168 -> [w1038]
          tunnel: w167 -> [w1023]
          tunnel: w166 -> [w1034]
          tunnel: [w1034] -> w189
          tunnel: w165 -> [w1025]
          tunnel: [w1025] -> w179
          tunnel: w164 -> [w1024]
          tunnel: [w1024] -> w177
          tunnel: [w1027] -> w153
          tunnel: w152 -> [w1027]
          tunnel: [w1028] -> w150
          tunnel: w149 -> [w1028]
          tunnel: [w1029] -> w147
          tunnel: w146 -> [w1029]
          tunnel: w145 -> [w1035]
          tunnel: [w1021] -> w112
          tunnel: w111 -> [w1021]
          tunnel: w231 -> [w1047]
          tunnel: w230 -> [w1064]
          tunnel: w227 -> [w1057]
          tunnel: w225 -> [w1063]
          tunnel: w223 -> [w1059]
          tunnel: w221 -> [w1062]
          tunnel: w219 -> [w1060]
          tunnel: w211 -> [w1061]
          tunnel: w189 -> [w1053]
          tunnel: w179 -> [w1052]
          tunnel: w177 -> [w1051]
          tunnel: w153 -> [w1050]
          tunnel: w150 -> [w1049]
          tunnel: w147 -> [w1048]
          tunnel: [w1046] -> w144
          tunnel: [w1064] -> w126
          tunnel: [w1057] -> w125
          tunnel: [w1063] -> w124
          tunnel: [w1059] -> w123
          tunnel: [w1062] -> w122
          tunnel: [w1060] -> w121
          tunnel: [w1061] -> w120
          tunnel: [w1053] -> w119
          tunnel: [w1052] -> w118
          tunnel: [w1051] -> w117
          tunnel: [w1050] -> w116
          tunnel: [w1049] -> w115
          tunnel: [w1048] -> w114
          tunnel: [w1045] -> w113
          tunnel: w112 -> [w1045]
          tunnel: w126 -> [w1100]
          tunnel: w125 -> [w1099]
          tunnel: w124 -> [w1098]
          tunnel: w123 -> [w1097]
          tunnel: w122 -> [w1096]
          tunnel: w121 -> [w1095]
          tunnel: w120 -> [w1094]
          tunnel: w119 -> [w1093]
          tunnel: w118 -> [w1092]
          tunnel: w117 -> [w1091]
          tunnel: w116 -> [w1090]
          tunnel: w115 -> [w1089]
          tunnel: w114 -> [w1088]
          tunnel: w113 -> [w1081]
          tunnel: [w1100] -> w106
          tunnel: [w1099] -> w105
          tunnel: [w1098] -> w104
          tunnel: [w1097] -> w103
          tunnel: [w1096] -> w102
          tunnel: [w1095] -> w101
          tunnel: [w1094] -> w100
          tunnel: [w1093] -> w99
          tunnel: [w1092] -> w98
          tunnel: [w1091] -> w97
          tunnel: [w1090] -> w96
          tunnel: [w1089] -> w95
          tunnel: [w1088] -> w94
          tunnel: [w1081] -> w93
          tunnel: [w1080] -> w92
          tunnel: [w1106] -> w148
          tunnel: [w1107] -> w151
          tunnel: [w1108] -> w154
          tunnel: [w1109] -> w178
          tunnel: [w1110] -> w180
          tunnel: [w1111] -> w190
          tunnel: [w1112] -> w212
          tunnel: [w1113] -> w220
          tunnel: [w1114] -> w222
          tunnel: [w1115] -> w224
          tunnel: [w1116] -> w226
          tunnel: [w1117] -> w228
          tunnel: [w1118] -> w229
          tunnel: w106 -> [w1118]
          tunnel: w105 -> [w1117]
          tunnel: w104 -> [w1116]
          tunnel: w103 -> [w1115]
          tunnel: w102 -> [w1114]
          tunnel: w101 -> [w1113]
          tunnel: w100 -> [w1112]
          tunnel: w99 -> [w1111]
          tunnel: w98 -> [w1110]
          tunnel: w97 -> [w1109]
          tunnel: w96 -> [w1108]
          tunnel: w95 -> [w1107]
          tunnel: w94 -> [w1106]
          tunnel: w93 -> [w1102]
          tunnel: w92 -> [w1101]
          frame #0 {
            n13 = Tick Count (ms)() -> (millisecond timer value=w251:u32)
          }
          frame #1 {
            n14 = while {
              tunnel: w281 -> [w289]
              tunnel: [w288] -> w280
              tunnel: [w287] -> w279
              tunnel: w275 -> [w286]
              tunnel: w274 -> [w285]
              stop <- w290 stop-if-true
              (unwired) "Daniel Schuster (geb. 20.03.1988)"
              n15 = event shown="[11] \"Write to File\": Value Change" {
                selector: _ -> [_ _ _ _ _ _ _ _ _ _ _ _]
                dyn-events: _ -> [_ _ _ _ _ _ _ _ _ _ _ _]
                timeout: 1 -> [_ _ _ _ _ _ _ _ _ _ _ _]
                tunnel: [TRUE ("Set Gauge to Zero") w298 w347 w368 w394 w429 w485 w536 w615 w686 "Set Gauge to Zero" _] -> w290
                tunnel: w289 -> [w294 w297 w344 w366 w390 w428 w481 w534 w613 w684 w763 w789]
                tunnel: [w293 w296 w343 w365 w392 w426 w483 w533 w612 w683 w762 w788] -> w288
                tunnel: [w292 w295 w342 w364 w391 w427 w482 w532 w611 w682 w761 w787] -> w287
                tunnel: w286 -> [_ _ _ _ _ _ _ _ _ _ w764 _]
                tunnel: w285 -> [_ _ _ _ _ _ _ _ _ _ w757 _]
                event Timeout {
                  n16 = event-data() -> ()  [unwired: 1 in, 1 out]
                  n17 = Unbundle(w294) -> ("VISA resource name out"=w293:refnum<visa-resource-name>, "error out"=w292:errorcluster)  [unwired: 2 out]
                }
                event "Setpoint\n START": Value Change {
                  n18 = event-data() -> ()  [unwired: 1 in, 1 out]
                  n19 = stacked-sequence {
                    tunnel: w297 -> [_ w304 _]
                    tunnel: [_ w303 _] -> w295
                    tunnel: [_ w302 _] -> w296
                    frame #0 {
                      n20 = property on="Setpoint\n START" class="Bool"("Blinking"=TRUE) -> ()  [unwired: 2 in, 2 out]
                      n21 = property on="Read Temperature" class="Bool (strict)"("Blinking"=FALSE) -> ()  [unwired: 2 in, 2 out]
                    }
                    frame #1 {
                      n22 = for {
                        N: 2 -> [_]
                        tunnel: w304 -> [w308]
                        tunnel: [w307] -> w303
                        tunnel: [w306] -> w302
                        i -> [w310]
                        n23 = flat-sequence {
                          tunnel: [w313] -> w309
                          tunnel: w310 -> [w312]
                          tunnel: [w331] -> w311
                          tunnel: w309 -> [w330]
                          tunnel: w308 -> [w332]
                          tunnel: [w329] -> w307
                          tunnel: [w328] -> w306
                          tunnel: w311 -> [w338]
                          tunnel: w310 -> [w337]
                          frame #0 {
                            n24 = case shown="0, Default" w312 {
                              tunnel: [w322 w324] -> w313
                              frame 0, Default {
                                n25 = Multiply(x=10.0, y="SP 1 shall be (°C)") -> (x*y=w319:dbl)
                                n26 = local read "RAM"() -> (w317:bool)
                                n27 = Number To Hexadecimal String(1:i16 5 ("width (-)"), 2:w319) -> (0:w321:string)
                                n28 = Select(t="*P012", s=w317, f="*P012") -> (s? t:f=w314:string)
                                n29 = Concatenate Strings(w314, w321) -> (w322:string)
                              }
                              frame 1 {
                                n30 = local read "RAM"() -> (w327:bool)
                                n31 = Select(t="*G01", s=w327, f="*R01") -> (s? t:f=w324:string)
                              }
                            }
                          }
                          frame #1 {
                            n32 = Unbundle(w332) -> ("VISA resource name out"=w333:refnum<visa-resource-name>, "error out"=w335:errorcluster, "Delay (ms)"=w334:u32, "Write/\nRead"=w336:bool)
                            n33 = call "I3252_Comm_Interface.vi"("VISA resource name in"=w333, "error in"=w335, "Delay (ms)"=w334, "Write"=w336, "String to Write"=w330, "Read"=w336) -> ("VISA resource name out"=w328:refnum<visa-resource-name>, "error out"=w329:errorcluster, "Read String"=w331:string)  [unwired: 2 in]
                          }
                          frame #2 {
                            n34 = case shown="0, Default" w337 {
                              tunnel: w338 -> [_ w340]
                              frame 0, Default {
                              }
                              frame 1 {
                                n35 = call "I3252_Edit_Setpoint.vi"("Read String"=w340) -> ("Setpoint is"=→"SP 1 is (°C)":dbl)
                              }
                            }
                          }
                        }
                      }
                    }
                    frame #2 {
                      n36 = property on="Setpoint\n START" class="Bool"("Blinking"=FALSE) -> ()  [unwired: 2 in, 2 out]
                    }
                  }
                  n37 = Not(x="Setpoint\n START") -> (.not. x?=w298:bool)
                }
                event "Standby": Value Change {
                  n38 = event-data() -> ()  [unwired: 1 in, 1 out]
                  n39 = flat-sequence {
                    tunnel: [w355] -> w345
                    tunnel: w345 -> [w359]
                    tunnel: w344 -> [w358]
                    tunnel: [w357] -> w342
                    tunnel: [w356] -> w343
                    frame #0 {
                      n40 = local read "Standby"() -> (w348:bool)
                      n41 = Select(t=TRUE, s=w348, f=FALSE) -> (s? t:f=w351:bool)
                      n42 = property on="Standby" class="Bool (strict)"("Blinking"=w351) -> ()  [unwired: 2 in, 2 out]
                    }
                    frame #1 {
                      n43 = local read "Standby"() -> (w353:bool)
                      n44 = Select(t="*D03", s=w353, f="*E03") -> (s? t:f=w355:string)
                    }
                    frame #2 {
                      n45 = Unbundle(w358) -> ("VISA resource name out"=w360:refnum<visa-resource-name>, "error out"=w362:errorcluster, "Delay (ms)"=w361:u32, "Write/\nRead"=w363:bool)
                      n46 = call "I3252_Comm_Interface.vi"("VISA resource name in"=w360, "error in"=w362, "Delay (ms)"=w361, "Write"=w363, "String to Write"=w359, "Read"=w363) -> ("VISA resource name out"=w356:refnum<visa-resource-name>, "error out"=w357:errorcluster)  [unwired: 2 in, 1 out]
                    }
                  }
                  n47 = Not(x="Standby") -> (.not. x?=w347:bool)
                }
                event "Set Command": Value Change {
                  n48 = event-data() -> ()  [unwired: 1 in, 1 out]
                  n49 = stacked-sequence {
                    tunnel: w366 -> [_ w373 _]
                    tunnel: [_ w372 _] -> w365
                    tunnel: [_ w371 _] -> w364
                    frame #0 {
                      n50 = property on="Set Command" class="Bool"("Blinking"=TRUE) -> ()  [unwired: 2 in, 2 out]
                      n51 = property on="Read Temperature" class="Bool (strict)"("Blinking"=FALSE) -> ()  [unwired: 2 in, 2 out]
                    }
                    frame #1 {
                      n52 = flat-sequence {
                        tunnel: [w378] -> w375
                        tunnel: [w381] -> w374
                        tunnel: w375 -> [w382]
                        tunnel: w373 -> [w383]
                        tunnel: [w380] -> w372
                        tunnel: [w379] -> _
                        tunnel: [w379] -> w371
                        tunnel: w374 -> [w388]
                        frame #0 {
                          n53 = Concatenate Strings("*", "Command shall be") -> (w378:string)
                        }
                        frame #1 {
                          n54 = Unbundle(w383) -> ("VISA resource name out"=w387:refnum<visa-resource-name>, "error out"=w385:errorcluster, "Delay (ms)"=w386:u32, "Write/\nRead"=w384:bool)
                          n55 = call "I3252_Comm_Interface.vi"("VISA resource name in"=w387, "error in"=w385, "Delay (ms)"=w386, "Write"=w384, "String to Write"=w382, "Read"=w384) -> ("VISA resource name out"=w380:refnum<visa-resource-name>, "error out"=w379:errorcluster, "Read String"=w381:string)  [unwired: 2 in]
                        }
                        frame #2 {
                          "Command is" <- w388
                        }
                      }
                    }
                    frame #2 {
                      n56 = property on="Set Command" class="Bool"("Blinking"=FALSE) -> ()  [unwired: 2 in, 2 out]
                    }
                  }
                  n57 = Not(x="Set Command") -> (.not. x?=w368:bool)
                }
                event "Reset\nSTOPP": Value Change {
                  n58 = event-data() -> ()  [unwired: 1 in, 1 out]
                  n59 = stacked-sequence {
                    tunnel: [_ w401 _] -> w391
                    tunnel: [_ w400 _] -> w392
                    tunnel: w390 -> [_ w398 _]
                    frame #0 {
                      n60 = property on="Reset\nSTOPP" class="Bool"("Blinking"=TRUE) -> ()  [unwired: 2 in, 2 out]
                      n61 = property on="Read Temperature" class="Bool (strict)"("Blinking"=FALSE) -> ()  [unwired: 2 in, 2 out]
                    }
                    frame #1 {
                      n62 = for {
                        N: 2 -> [_]
                        tunnel: [w407] -> w401
                        tunnel: [w406] -> w400
                        tunnel: w398 -> [w405]
                        i -> [w403]
                        n63 = flat-sequence {
                          tunnel: w403 -> [w409]
                          tunnel: [w408] -> w404
                          tunnel: [w414] -> w407
                          tunnel: [w415] -> w406
                          tunnel: w405 -> [w416]
                          tunnel: w404 -> [w413]
                          tunnel: [w412] -> w402
                          tunnel: w403 -> [w422]
                          tunnel: w402 -> [w421]
                          frame #0 {
                            n64 = case shown="0, Default" w409 {
                              tunnel: ["*Z02" "*G01"] -> w408
                              frame 0, Default {
                              }
                              frame 1 {
                              }
                            }
                          }
                          frame #1 {
                            n65 = Unbundle(w416) -> ("VISA resource name out"=w417:refnum<visa-resource-name>, "error out"=w419:errorcluster, "Delay (ms)"=w418:u32, "Write/\nRead"=w420:bool)
                            n66 = call "I3252_Comm_Interface.vi"("VISA resource name in"=w417, "error in"=w419, "Delay (ms)"=w418, "Write"=w420, "String to Write"=w413, "Read"=w420) -> ("VISA resource name out"=w415:refnum<visa-resource-name>, "error out"=w414:errorcluster, "Read String"=w412:string)  [unwired: 2 in]
                          }
                          frame #2 {
                            n67 = case shown="0, Default" w422 {
                              tunnel: w421 -> [_ w424]
                              frame 0, Default {
                              }
                              frame 1 {
                                n68 = call "I3252_Edit_Setpoint.vi"("Read String"=w424) -> ("Setpoint is"=w423:dbl)
                                n69 = local write "SP 1 is (°C)"(w423) -> ()
                              }
                            }
                          }
                        }
                      }
                      n70 = Wait (ms)(milliseconds to wait=u32 4000) -> ()  [unwired: 1 out]
                    }
                    frame #2 {
                      n71 = property on="Reset\nSTOPP" class="Bool"("Blinking"=FALSE) -> ()  [unwired: 2 in, 2 out]
                    }
                  }
                  n72 = Not(x="Reset\nSTOPP") -> (.not. x?=w394:bool)
                }
                event "Auto Tune": Value Change {
                  n73 = event-data() -> ()  [unwired: 1 in, 1 out]
                  n74 = stacked-sequence {
                    tunnel: w428 -> [_ w435 w480]
                    tunnel: [_ w434 _] -> w427
                    tunnel: [_ w433 _] -> w426
                    frame #0 {
                      n75 = property on="Auto Tune" class="Bool"("Blinking"=TRUE) -> ()  [unwired: 2 in, 2 out]
                      n76 = property on="Read Temperature" class="Bool (strict)"("Blinking"=FALSE) -> ()  [unwired: 2 in, 2 out]
                    }
                    frame #1 {
                      n77 = for {
                        N: 4 -> [_]
                        tunnel: [w440] -> w433
                        tunnel: [w439] -> w434
                        tunnel: w435 -> [w438]
                        i -> [w443]
                        n78 = flat-sequence {
                          tunnel: w443 -> [w445]
                          tunnel: [w444] -> w441
                          tunnel: w441 -> [w460]
                          tunnel: [w459] -> w442
                          tunnel: [w462] -> w440
                          tunnel: [w461] -> w439
                          tunnel: w438 -> [w458]
                          tunnel: w443 -> [w468]
                          tunnel: w442 -> [w467]
                          frame #0 {
                            n79 = case shown="0, Default" w445 {
                              tunnel: ["*V01" w448 "*W0C35" "*Z02"] -> w444
                              frame 0, Default {
                              }
                              frame 1 {
                                n80 = local read "Temperature (°C)"() -> (w447:dbl)
                                n81 = Add(x=20.0, y=w447) -> (x+y=w454:dbl)
                                n82 = Multiply(x=10.0, y=w454) -> (x*y=w451:dbl)
                                n83 = Number To Hexadecimal String(1:i16 5 ("width (-)"), 2:w451) -> (0:w450:string)
                                n84 = Concatenate Strings("*W012", w450) -> (w448:string)
                              }
                              frame 2 {
                                # "35 hex = \n00110101 bin"
                              }
                              frame 3 {
                              }
                            }
                          }
                          frame #1 {
                            n85 = Unbundle(w458) -> ("VISA resource name out"=w466:refnum<visa-resource-name>, "error out"=w464:errorcluster, "Delay (ms)"=w465:u32, "Write/\nRead"=w463:bool)
                            n86 = call "I3252_Comm_Interface.vi"("VISA resource name in"=w466, "error in"=w464, "Delay (ms)"=w465, "Write"=w463, "String to Write"=w460, "Read"=w463) -> ("VISA resource name out"=w462:refnum<visa-resource-name>, "error out"=w461:errorcluster, "Read String"=w459:string)  [unwired: 2 in]
                          }
                          frame #2 {
                            n87 = case shown="0, Default" w468 {
                              tunnel: w467 -> [w470]
                              frame 0, Default {
                                n88 = call <vilib>:"Space Constant.vi"() -> ("String"=w473:string)
                                n89 = Search/Split String(string=w470, search string/char (-)=w473) -> (match + rest of string=w472:string)  [unwired: 1 in, 2 out]
                                n90 = Fract/Exp String To Number(use system decimal point (T)=FALSE, string=w472) -> (number=w469:dbl)  [unwired: 2 in, 1 out]
                                n91 = local write "Temperature (°C)"(w469) -> ()
                              }
                            }
                          }
                        }
                      }
                      n92 = Wait (ms)(milliseconds to wait=u32 45000) -> ()  [unwired: 1 out]
                    }
                    frame #2 {
                      n93 = Unbundle(w480) -> ("VISA resource name out"=w479:refnum<visa-resource-name>, "error out"=w477:errorcluster, "Delay (ms)"=w478:u32, "Write/\nRead"=w476:bool)
                      n94 = property on="Auto Tune" class="Bool"("Blinking"=FALSE) -> ()  [unwired: 2 in, 2 out]
                      n95 = call "I3252_Comm_Interface.vi"("VISA resource name in"=w479, "error in"=w477, "Delay (ms)"=w478, "Write"=w476, "String to Write"="*W01200000", "Read"=w476) -> ()  [unwired: 2 in, 3 out]
                    }
                  }
                  n96 = Not(x="Auto Tune") -> (.not. x?=w429:bool)
                }
                event "Write LOW/HI": Value Change {
                  n97 = event-data() -> ()  [unwired: 1 in, 1 out]
                  n98 = stacked-sequence {
                    tunnel: [_ w490 _] -> w483
                    tunnel: [_ w489 _] -> w482
                    tunnel: w481 -> [_ w488 _]
                    frame #0 {
                      n99 = property on="Write LOW/HI" class="Bool"("Blinking"=TRUE) -> ()  [unwired: 2 in, 2 out]
                      n100 = property on="Read Temperature" class="Bool (strict)"("Blinking"=FALSE) -> ()  [unwired: 2 in, 2 out]
                    }
                    frame #1 {
                      n101 = for {
                        N: 4 -> [_]
                        tunnel: [w494] -> w490
                        tunnel: [w493] -> w489
                        tunnel: w488 -> [w492]
                        i -> [w496]
                        n102 = flat-sequence {
                          tunnel: w496 -> [w498]
                          tunnel: [w499] -> w495
                          tunnel: w495 -> [w513]
                          tunnel: [w514] -> w497
                          tunnel: [w516] -> w494
                          tunnel: [w515] -> w493
                          tunnel: w492 -> [w512]
                          tunnel: w497 -> [w522]
                          tunnel: w496 -> [w521]
                          frame #0 {
                            n103 = case shown="1" w498 {
                              tunnel: [w501 w507 "*R27" "*R28"] -> w499
                              frame 0, Default {
                                n104 = Number To Hexadecimal String(1:i16 2 ("width (-)"), 2:"% LOW shall be") -> (0:w502:string)
                                n105 = Concatenate Strings("*W27", w502) -> (w501:string)
                              }
                              frame 1 {
                                n106 = Number To Hexadecimal String(1:i16 2 ("width (-)"), 2:"% High shall be") -> (0:w508:string)
                                n107 = Concatenate Strings("*W28", w508) -> (w507:string)
                              }
                              frame 2 {
                              }
                              frame 3 {
                              }
                            }
                          }
                          frame #1 {
                            n108 = Unbundle(w512) -> ("VISA resource name out"=w520:refnum<visa-resource-name>, "error out"=w518:errorcluster, "Delay (ms)"=w519:u32, "Write/\nRead"=w517:bool)
                            n109 = call "I3252_Comm_Interface.vi"("VISA resource name in"=w520, "error in"=w518, "Delay (ms)"=w519, "Write"=w517, "String to Write"=w513, "Read"=w517) -> ("VISA resource name out"=w516:refnum<visa-resource-name>, "error out"=w515:errorcluster, "Read String"=w514:string)  [unwired: 2 in]
                          }
                          frame #2 {
                            n110 = case shown="0, Default" w521 {
                              tunnel: w522 -> [_ w526 w530]
                              frame 0, Default {
                              }
                              frame 2 {
                                n111 = String Subset(string=w526, offset (0)=3) -> (substring=w524:string)  [unwired: 1 in]
                                n112 = Hexadecimal String To Number(string=w524) -> (number=→"% LOW is":u32)  [unwired: 2 in, 1 out]
                              }
                              frame 3 {
                                n113 = String Subset(string=w530, offset (0)=3) -> (substring=w528:string)  [unwired: 1 in]
                                n114 = Hexadecimal String To Number(string=w528) -> (number=→"% HIGH is":u32)  [unwired: 2 in, 1 out]
                              }
                            }
                          }
                        }
                      }
                    }
                    frame #2 {
                      n115 = property on="Write LOW/HI" class="Bool"("Blinking"=FALSE) -> ()  [unwired: 2 in, 2 out]
                    }
                  }
                  n116 = Not(x="Write LOW/HI") -> (.not. x?=w485:bool)
                }
                event "Set PID": Value Change {
                  n117 = event-data() -> ()  [unwired: 1 in, 1 out]
                  n118 = stacked-sequence {
                    tunnel: w534 -> [_ w541 _]
                    tunnel: [_ w540 _] -> w533
                    tunnel: [_ w539 _] -> w532
                    frame #0 {
                      n119 = property on="Set PID" class="Bool"("Blinking"=TRUE) -> ()  [unwired: 2 in, 2 out]
                      n120 = property on="Read Temperature" class="Bool (strict)"("Blinking"=FALSE) -> ()  [unwired: 2 in, 2 out]
                    }
                    frame #1 {
                      n121 = for {
                        N: 6 -> [_]
                        tunnel: w541 -> [w545]
                        tunnel: [w544] -> w540
                        tunnel: [w543] -> w539
                        i -> [w547]
                        n122 = flat-sequence {
                          tunnel: w547 -> [w549]
                          tunnel: [w550] -> w546
                          tunnel: w546 -> [w591]
                          tunnel: [w587] -> w548
                          tunnel: w545 -> [w590]
                          tunnel: [w589] -> w543
                          tunnel: [w588] -> w544
                          tunnel: w548 -> [w597]
                          tunnel: w547 -> [w596]
                          frame #0 {
                            n123 = case shown="0, Default" w549 {
                              tunnel: [w557 w565 w573 w575 w579 w583] -> w550
                              frame 0, Default {
                                n124 = local read "RAM"() -> (w551:bool)
                                n125 = Number To Hexadecimal String(1:i16 4 ("width (-)"), 2:"P (PB1) shall be") -> (0:w558:string)
                                n126 = Select(t="*P17", s=w551, f="*W17") -> (s? t:f=w552:string)
                                n127 = Concatenate Strings(w552, w558) -> (w557:string)
                              }
                              frame 1 {
                                n128 = local read "RAM"() -> (w559:bool)
                                n129 = Number To Hexadecimal String(1:i16 4 ("width (-)"), 2:"I ( Reset1) shall be") -> (0:w566:string)
                                n130 = Select(t="*P18", s=w559, f="*W18") -> (s? t:f=w561:string)
                                n131 = Concatenate Strings(w561, w566) -> (w565:string)
                              }
                              frame 2 {
                                n132 = local read "RAM"() -> (w568:bool)
                                n133 = Number To Hexadecimal String(1:i16 4 ("width (-)"), 2:"D (Rate) shall be") -> (0:w574:string)
                                n134 = Select(t="*P19", s=w568, f="*W19") -> (s? t:f=w569:string)
                                n135 = Concatenate Strings(w569, w574) -> (w573:string)
                              }
                              frame 3 {
                                n136 = local read "RAM"() -> (w578:bool)
                                n137 = Select(t="*G17", s=w578, f="*R17") -> (s? t:f=w575:string)
                              }
                              frame 4 {
                                n138 = local read "RAM"() -> (w582:bool)
                                n139 = Select(t="*G18", s=w582, f="*R18") -> (s? t:f=w579:string)
                              }
                              frame 5 {
                                n140 = local read "RAM"() -> (w586:bool)
                                n141 = Select(t="*G19", s=w586, f="*R19") -> (s? t:f=w583:string)
                              }
                            }
                          }
                          frame #1 {
                            n142 = Unbundle(w590) -> ("VISA resource name out"=w595:refnum<visa-resource-name>, "error out"=w593:errorcluster, "Delay (ms)"=w594:u32, "Write/\nRead"=w592:bool)
                            n143 = call "I3252_Comm_Interface.vi"("VISA resource name in"=w595, "error in"=w593, "Delay (ms)"=w594, "Write"=w592, "String to Write"=w591, "Read"=w592) -> ("VISA resource name out"=w588:refnum<visa-resource-name>, "error out"=w589:errorcluster, "Read String"=w587:string)  [unwired: 2 in]
                          }
                          frame #2 {
                            n144 = case shown="0, Default" w596 {
                              tunnel: w597 -> [_ w601 w605 w609]
                              frame 0, Default {
                              }
                              frame 3 {
                                n145 = String Subset(string=w601, offset (0)=3) -> (substring=w599:string)  [unwired: 1 in]
                                n146 = Hexadecimal String To Number(string=w599) -> (number=→"P (PB1) is":u32)  [unwired: 2 in, 1 out]
                              }
                              frame 4 {
                                n147 = String Subset(string=w605, offset (0)=3) -> (substring=w603:string)  [unwired: 1 in]
                                n148 = Hexadecimal String To Number(string=w603) -> (number=→"I ( Reset1) is":u32)  [unwired: 2 in, 1 out]
                              }
                              frame 5 {
                                n149 = String Subset(string=w609, offset (0)=3) -> (substring=w607:string)  [unwired: 1 in]
                                n150 = Hexadecimal String To Number(string=w607) -> (number=→"D (Rate) is":u32)  [unwired: 2 in, 1 out]
                              }
                            }
                          }
                        }
                      }
                    }
                    frame #2 {
                      n151 = property on="Set PID" class="Bool"("Blinking"=FALSE) -> ()  [unwired: 2 in, 2 out]
                    }
                  }
                  n152 = Not(x="Set PID") -> (.not. x?=w536:bool)
                }
                event "Get Values": Value Change {
                  n153 = event-data() -> ()  [unwired: 1 in, 1 out]
                  n154 = stacked-sequence {
                    tunnel: w613 -> [_ w620 _]
                    tunnel: [_ w619 _] -> w612
                    tunnel: [_ w618 _] -> w611
                    frame #0 {
                      n155 = property on="Get Values" class="Bool"("Blinking"=TRUE) -> ()  [unwired: 2 in, 2 out]
                      n156 = property on="Read Temperature" class="Bool (strict)"("Blinking"=FALSE) -> ()  [unwired: 2 in, 2 out]
                    }
                    frame #1 {
                      n157 = for {
                        N: 6 -> [_]
                        tunnel: w620 -> [w624]
                        tunnel: [w623] -> w619
                        tunnel: [w622] -> w618
                        i -> [w626]
                        n158 = flat-sequence {
                          tunnel: w626 -> [w628]
                          tunnel: [w629] -> w625
                          tunnel: w625 -> [w651]
                          tunnel: [w652] -> w627
                          tunnel: w624 -> [w650]
                          tunnel: [w649] -> w622
                          tunnel: [w648] -> w623
                          tunnel: w627 -> [w658]
                          tunnel: w626 -> [w657]
                          frame #0 {
                            n159 = case shown="0, Default" w628 {
                              tunnel: [w632 w636 w640 "*R27" "*R28" w646] -> w629
                              frame 0, Default {
                                n160 = local read "RAM"() -> (w633:bool)
                                n161 = Select(t="*G17", s=w633, f="*R17") -> (s? t:f=w632:string)
                              }
                              frame 1 {
                                n162 = local read "RAM"() -> (w637:bool)
                                n163 = Select(t="*G18", s=w637, f="*R18") -> (s? t:f=w636:string)
                              }
                              frame 2 {
                                n164 = local read "RAM"() -> (w641:bool)
                                n165 = Select(t="*G19", s=w641, f="*R19") -> (s? t:f=w640:string)
                              }
                              frame 3 {
                              }
                              frame 4 {
                              }
                              frame 5 {
                                n166 = local read "RAM"() -> (w647:bool)
                                n167 = Select(t="*G01", s=w647, f="*R01") -> (s? t:f=w646:string)
                              }
                            }
                          }
                          frame #1 {
                            n168 = Unbundle(w650) -> ("VISA resource name out"=w656:refnum<visa-resource-name>, "error out"=w654:errorcluster, "Delay (ms)"=w655:u32, "Write/\nRead"=w653:bool)
                            n169 = call "I3252_Comm_Interface.vi"("VISA resource name in"=w656, "error in"=w654, "Delay (ms)"=w655, "Write"=w653, "String to Write"=w651, "Read"=w653) -> ("VISA resource name out"=w648:refnum<visa-resource-name>, "error out"=w649:errorcluster, "Read String"=w652:string)  [unwired: 2 in]
                          }
                          frame #2 {
                            n170 = case shown="0, Default" w657 {
                              tunnel: w658 -> [w660 w664 w668 w672 w676 w680]
                              frame 0, Default {
                                n171 = String Subset(string=w660, offset (0)=3) -> (substring=w661:string)  [unwired: 1 in]
                                n172 = Hexadecimal String To Number(string=w661) -> (number=w659:u32)  [unwired: 2 in, 1 out]
                                n173 = local write "P (PB1) shall be"(w659) -> ()
                                n174 = local write "P (PB1) is"(w659) -> ()
                              }
                              frame 1 {
                                n175 = String Subset(string=w664, offset (0)=3) -> (substring=w665:string)  [unwired: 1 in]
                                n176 = Hexadecimal String To Number(string=w665) -> (number=w663:u32)  [unwired: 2 in, 1 out]
                                n177 = local write "I ( Reset1) shall be"(w663) -> ()
                                n178 = local write "I ( Reset1) is"(w663) -> ()
                              }
                              frame 2 {
                                n179 = String Subset(string=w668, offset (0)=3) -> (substring=w669:string)  [unwired: 1 in]
                                n180 = Hexadecimal String To Number(string=w669) -> (number=w667:u32)  [unwired: 2 in, 1 out]
                                n181 = local write "D (Rate) shall be"(w667) -> ()
                                n182 = local write "D (Rate) is"(w667) -> ()
                              }
                              frame 3 {
                                n183 = String Subset(string=w672, offset (0)=3) -> (substring=w673:string)  [unwired: 1 in]
                                n184 = Hexadecimal String To Number(string=w673) -> (number=w671:u32)  [unwired: 2 in, 1 out]
                                n185 = local write "% LOW shall be"(w671) -> ()
                                n186 = local write "% LOW is"(w671) -> ()
                              }
                              frame 4 {
                                n187 = String Subset(string=w676, offset (0)=3) -> (substring=w677:string)  [unwired: 1 in]
                                n188 = Hexadecimal String To Number(string=w677) -> (number=w675:u32)  [unwired: 2 in, 1 out]
                                n189 = local write "% High shall be"(w675) -> ()
                                n190 = local write "% HIGH is"(w675) -> ()
                              }
                              frame 5 {
                                n191 = call "I3252_Edit_Setpoint.vi"("Read String"=w680) -> ("Setpoint is"=w679:dbl)
                                n192 = local write "SP 1 is (°C)"(w679) -> ()
                              }
                            }
                          }
                        }
                      }
                    }
                    frame #2 {
                      n193 = property on="Get Values" class="Bool"("Blinking"=FALSE) -> ()  [unwired: 2 in, 2 out]
                    }
                  }
                  n194 = Not(x="Get Values") -> (.not. x?=w615:bool)
                }
                event "RAM": Value Change {
                  n195 = event-data() -> ()  [unwired: 1 in, 1 out]
                  n196 = stacked-sequence {
                    tunnel: w684 -> [_ w691 _]
                    tunnel: [_ w690 _] -> w683
                    tunnel: [_ w689 _] -> w682
                    frame #0 {
                      n197 = property on="RAM" class="Bool (strict)"("Blinking"=TRUE) -> ()  [unwired: 2 in, 2 out]
                      n198 = property on="Read Temperature" class="Bool (strict)"("Blinking"=FALSE) -> ()  [unwired: 2 in, 2 out]
                    }
                    frame #1 {
                      n199 = for {
                        N: 6 -> [_]
                        tunnel: w691 -> [w695]
                        tunnel: [w694] -> w690
                        tunnel: [w693] -> w689
                        i -> [w697]
                        n200 = flat-sequence {
                          tunnel: w697 -> [w699]
                          tunnel: [w700] -> w696
                          tunnel: w696 -> [w719]
                          tunnel: [w720] -> w698
                          tunnel: w695 -> [w723]
                          tunnel: [w722] -> w693
                          tunnel: [w721] -> w694
                          tunnel: w698 -> [w729]
                          tunnel: w697 -> [w728]
                          frame #0 {
                            n201 = case shown="0, Default" w699 {
                              tunnel: [w703 w707 w711 "*R27" "*R28" w717] -> w700
                              frame 0, Default {
                                n202 = local read "RAM"() -> (w704:bool)
                                n203 = Select(t="*G17", s=w704, f="*R17") -> (s? t:f=w703:string)
                              }
                              frame 1 {
                                n204 = local read "RAM"() -> (w708:bool)
                                n205 = Select(t="*G18", s=w708, f="*R18") -> (s? t:f=w707:string)
                              }
                              frame 2 {
                                n206 = local read "RAM"() -> (w712:bool)
                                n207 = Select(t="*G19", s=w712, f="*R19") -> (s? t:f=w711:string)
                              }
                              frame 3 {
                              }
                              frame 4 {
                              }
                              frame 5 {
                                n208 = local read "RAM"() -> (w718:bool)
                                n209 = Select(t="*G01", s=w718, f="*R01") -> (s? t:f=w717:string)
                              }
                            }
                          }
                          frame #1 {
                            n210 = Unbundle(w723) -> ("VISA resource name out"=w727:refnum<visa-resource-name>, "error out"=w725:errorcluster, "Delay (ms)"=w726:u32, "Write/\nRead"=w724:bool)
                            n211 = call "I3252_Comm_Interface.vi"("VISA resource name in"=w727, "error in"=w725, "Delay (ms)"=w726, "Write"=w724, "String to Write"=w719, "Read"=w724) -> ("VISA resource name out"=w721:refnum<visa-resource-name>, "error out"=w722:errorcluster, "Read String"=w720:string)  [unwired: 2 in]
                          }
                          frame #2 {
                            n212 = case shown="0, Default" w728 {
                              tunnel: w729 -> [w731 w735 w739 w743 w747 w751]
                              frame 0, Default {
                                n213 = String Subset(string=w731, offset (0)=3) -> (substring=w732:string)  [unwired: 1 in]
                                n214 = Hexadecimal String To Number(string=w732) -> (number=w730:u32)  [unwired: 2 in, 1 out]
                                n215 = local write "P (PB1) shall be"(w730) -> ()
                                n216 = local write "P (PB1) is"(w730) -> ()
                              }
                              frame 1 {
                                n217 = String Subset(string=w735, offset (0)=3) -> (substring=w736:string)  [unwired: 1 in]
                                n218 = Hexadecimal String To Number(string=w736) -> (number=w734:u32)  [unwired: 2 in, 1 out]
                                n219 = local write "I ( Reset1) shall be"(w734) -> ()
                                n220 = local write "I ( Reset1) is"(w734) -> ()
                              }
                              frame 2 {
                                n221 = String Subset(string=w739, offset (0)=3) -> (substring=w740:string)  [unwired: 1 in]
                                n222 = Hexadecimal String To Number(string=w740) -> (number=w738:u32)  [unwired: 2 in, 1 out]
                                n223 = local write "D (Rate) shall be"(w738) -> ()
                                n224 = local write "D (Rate) is"(w738) -> ()
                              }
                              frame 3 {
                                n225 = String Subset(string=w743, offset (0)=3) -> (substring=w744:string)  [unwired: 1 in]
                                n226 = Hexadecimal String To Number(string=w744) -> (number=w742:u32)  [unwired: 2 in, 1 out]
                                n227 = local write "% LOW shall be"(w742) -> ()
                                n228 = local write "% LOW is"(w742) -> ()
                              }
                              frame 4 {
                                n229 = String Subset(string=w747, offset (0)=3) -> (substring=w748:string)  [unwired: 1 in]
                                n230 = Hexadecimal String To Number(string=w748) -> (number=w746:u32)  [unwired: 2 in, 1 out]
                                n231 = local write "% High shall be"(w746) -> ()
                                n232 = local write "% HIGH is"(w746) -> ()
                              }
                              frame 5 {
                                n233 = call "I3252_Edit_Setpoint.vi"("Read String"=w751) -> ("Setpoint is"=w750:dbl)
                                n234 = local write "SP 1 is (°C)"(w750) -> ()
                              }
                            }
                          }
                        }
                      }
                    }
                    frame #2 {
                      n235 = property on="RAM" class="Bool (strict)"("Blinking"=FALSE) -> ()  [unwired: 2 in, 2 out]
                    }
                  }
                  n236 = Not(x="RAM") -> (.not. x?=w686:bool)
                }
                event "Set Gauge to Zero": Value Change {
                  n237 = event-data() -> ()  [unwired: 1 in, 1 out]
                  n238 = flat-sequence {
                    tunnel: w757 -> [w766]
                    tunnel: w764 -> [w767]
                    tunnel: w757 -> [w768]
                    tunnel: [w768] -> w755
                    tunnel: [w767] -> w754
                    tunnel: [w766] -> w753
                    tunnel: [w770] -> w760
                    tunnel: [w769] -> w759
                    tunnel: [w771] -> w758
                    tunnel: w755 -> [w773]
                    tunnel: w754 -> [w772]
                    tunnel: w753 -> [w771]
                    tunnel: w760 -> [w778]
                    tunnel: w759 -> [w777]
                    tunnel: w758 -> [w776]
                    frame #0 {
                      n239 = property on="Set Gauge to Zero" class="Bool"("Blinking"=TRUE) -> ()  [unwired: 2 in, 2 out]
                    }
                    frame #1 {
                      n240 = call "Pfeiffer_Get_Pressure_Status.vi"("Port"=w773, "Sensor Nr.:"=w772) -> ("Pressure"=w770:dbl)  [unwired: 1 in, 8 out]
                      "Pressure 2 (mbar)" <- w770
                      n241 = call "Pfeiffer_Offset_Display.vi"("Port"=w773, "W/R"=FALSE) -> ("Sensor 1 Get"=w769:dbl)  [unwired: 3 in, 6 out]
                      "Old Offset (mbar)" <- w769
                    }
                    frame #2 {
                      n242 = Add(x=w778, y=w777) -> (x+y=w780:dbl)
                      n243 = call "Pfeiffer_Offset_Display.vi"("Port"=w776, "W/R"=TRUE, "Sensor 1 Set"=w780) -> ("Sensor 1 Get"=→"Current Offset (mbar)":dbl)  [unwired: 2 in, 6 out]
                    }
                    frame #3 {
                      n244 = property on="Set Gauge to Zero" class="Bool"("Blinking"=TRUE) -> ()  [unwired: 2 in, 2 out]
                    }
                  }
                  n245 = Unbundle(w763) -> ("VISA resource name out"=w762:refnum<visa-resource-name>, "error out"=w761:errorcluster)  [unwired: 2 out]
                }
                event "Write to File": Value Change {
                  n246 = event-data() -> ("NewVal"=w786:bool)  [unwired: 1 in]
                  n247 = Unbundle(w789) -> ("VISA resource name out"=w788:refnum<visa-resource-name>, "error out"=w787:errorcluster)  [unwired: 2 out]
                  n248 = local read "File Path"() -> (w782:path)
                  n249 = case shown="True" w786 {
                    tunnel: w782 -> [_ w794]
                    tunnel: "User" -> [_ w793]
                    tunnel: "Sample" -> [_ w792]
                    tunnel: [path "" ("File Path") w791] -> w783
                    frame False {
                    }
                    frame True {
                      n250 = call "Header.vi"("Sample"=w792, "User"=w793, "File Path"=w794) -> ("File Path"=w791:path)
                    }
                  }
                  n251 = local write "File Path"(w783) -> ()
                }
              }
            }
            n252 = Bundle(cluster=w281, "VISA resource name out"=w280, "error out"=w279) -> (w278:T9)  [unwired: 2 in]
          }
          frame #2 {
          }
          frame #3 {
            (unwired) "Daniel Schuster (geb. 20.03.1988)"
            n253 = node-c288(w846) -> (w849:T5)  [unwired: 2 in]
            n254 = node-c288(w833) -> (w835:T5)  [unwired: 2 in]
            n255 = node-c288(w828) -> (w838:T5)  [unwired: 2 in]
            n256 = node-c288(w845) -> (w853:T5)  [unwired: 2 in]
            n257 = timed-sequence {
              timing: w849 -> [_]
              timing-out: [_] -> w848
              tunnel: w847 -> [w919]
              tunnel: [w918] -> w842
              tunnel: [w917] -> w841
              tunnel: [w916] -> w824
              n258 = timed-flat-sequence {
                tunnel: w919 -> [w923]
                tunnel: [w922] -> w918
                tunnel: [w921] -> w917
                tunnel: [w920] -> w916
                n259 = node-c288() -> ()  [unwired: 1 in, 1 out]
                n260 = case shown="True" "Read Temperature" {
                  tunnel: w923 -> [w927 w932]
                  tunnel: [w926 w931] -> w922
                  tunnel: [w925 w930] -> w921
                  tunnel: [_ w929] -> w920
                  frame False {
                    n261 = Unbundle(w927) -> ("VISA resource name out"=w926:refnum<visa-resource-name>, "error out"=w925:errorcluster)  [unwired: 2 out]
                    n262 = property on="Read Temperature" class="Bool (strict)"("Blinking"=FALSE) -> ()  [unwired: 2 in, 2 out]
                  }
                  frame True {
                    n263 = stacked-sequence {
                      tunnel: w932 -> [_ w937]
                      tunnel: [_ w936] -> w931
                      tunnel: [_ w935] -> w930
                      tunnel: [_ w934] -> w929
                      frame #0 {
                        n264 = property on="Read Temperature" class="Bool (strict)"("Blinking"=TRUE) -> ()  [unwired: 2 in, 2 out]
                      }
                      frame #1 {
                        n265 = Unbundle(w937) -> ("VISA resource name out"=w941:refnum<visa-resource-name>, "error out"=w939:errorcluster, "Delay (ms)"=w940:u32, "Write/\nRead"=w938:bool)
                        n266 = call "I3252_Comm_Interface.vi"("VISA resource name in"=w941, "error in"=w939, "Delay (ms)"=w940, "Write"=w938, "String to Write"="*V01", "Read"=w938) -> ("VISA resource name out"=w936:refnum<visa-resource-name>, "error out"=w935:errorcluster, "Read String"=w934:string)  [unwired: 2 in]
                      }
                    }
                  }
                }
                n267 = node-c288() -> ()  [unwired: 1 in, 1 out]
              }
            }
            n268 = timed-sequence {
              timing: w835 -> [_]
              timing-out: [_] -> w834
              tunnel: w832 -> [w858]
              tunnel: w831 -> [w857]
              tunnel: [w856] -> w829
              tunnel: [w855] -> w830
              tunnel: [w854] -> w826
              n269 = timed-flat-sequence {
                tunnel: w858 -> [w863]
                tunnel: w857 -> [w862]
                tunnel: [w861] -> w856
                tunnel: [w860] -> w855
                tunnel: [w859] -> w854
                n270 = node-c288() -> ()  [unwired: 1 in, 1 out]
                n271 = case shown="True" "Read VC 840 2" {
                  tunnel: w863 -> [w867 w873]
                  tunnel: w862 -> [w868 w872]
                  tunnel: [w867 w871] -> w861
                  tunnel: [w868 w870] -> w860
                  tunnel: [0.0 ("Reading") w869] -> w859
                  frame False {
                    n272 = property on="Read VC 840 2" class="Bool (strict)"("Blinking"=FALSE) -> ()  [unwired: 2 in, 2 out]
                  }
                  frame True {
                    n273 = stacked-sequence {
                      tunnel: w873 -> [_ w880]
                      tunnel: w872 -> [_ w879]
                      tunnel: [_ w878] -> w871
                      tunnel: [_ w877] -> w870
                      tunnel: [_ w875] -> w869
                      frame #0 {
                        n274 = property on="Read VC 840 2" class="Bool (strict)"("Blinking"=TRUE) -> ()  [unwired: 2 in, 2 out]
                      }
                      frame #1 {
                        n275 = call "VC840_Read.vi"("error in (no error)"=w879, "VISA resource name"=w880) -> ("error out"=w877:errorcluster, "Unit"=→"Unit 2":string, "Reading"=w875:dbl, "VISA resource name out"=w878:refnum<visa-resource-name>, "Status"=→"Status 2":T4, "Mode"=→"Mode 2":enum16{"?", "Diode", "Beep", "DC", "AC"})  [unwired: 4 out]
                        "Reading 2" <- w875
                      }
                    }
                  }
                }
                n276 = node-c288() -> ()  [unwired: 1 in, 1 out]
              }
            }
            n277 = timed-sequence {
              timing: w838 -> [_]
              timing-out: [_] -> w837
              tunnel: w840 -> [w892]
              tunnel: w839 -> [w891]
              tunnel: [w890] -> w836
              tunnel: [w889] -> w825
              n278 = timed-flat-sequence {
                tunnel: w892 -> [w896]
                tunnel: w891 -> [w895]
                tunnel: [w894] -> w890
                tunnel: [w893] -> w889
                n279 = node-c288() -> ()  [unwired: 1 in, 1 out]
                n280 = case shown="True" "Read Pressure" {
                  tunnel: w896 -> [_ w901]
                  tunnel: w895 -> [_ w902]
                  tunnel: [_ w903] -> w894
                  tunnel: [0.0 ("Pressure") w900] -> w893
                  frame False {
                    n281 = property on="Read Pressure" class="Bool (strict)"("Blinking"=FALSE) -> ()  [unwired: 2 in, 2 out]
                  }
                  frame True {
                    n282 = stacked-sequence {
                      tunnel: [_ w909] -> w903
                      tunnel: w902 -> [_ w908]
                      tunnel: w901 -> [_ w907]
                      tunnel: [_ w905] -> w900
                      frame #0 {
                        n283 = property on="Read Pressure" class="Bool (strict)"("Blinking"=TRUE) -> ()  [unwired: 2 in, 2 out]
                      }
                      frame #1 {
                        n284 = call "Pfeiffer_Get_Pressure_Status.vi"("Port"=w908, "Sensor Nr.:"=w907) -> ("Pressure"=w905:dbl, "Status"=→"Status":i32, "Error Out"=w909:bool)  [unwired: 7 in]
                        "Pressure 1 (mbar)" <- w905
                        "Pressure (mbar)" <- w905
                      }
                    }
                  }
                }
                n285 = node-c288() -> ()  [unwired: 1 in, 1 out]
              }
            }
            n286 = timed-sequence {
              timing: w853 -> [_]
              timing-out: [_] -> w852
              tunnel: w851 -> [w953]
              tunnel: w850 -> [w952]
              tunnel: [w951] -> w844
              tunnel: [w950] -> w843
              tunnel: [w949] -> w827
              n287 = timed-flat-sequence {
                tunnel: w953 -> [w958]
                tunnel: w952 -> [w957]
                tunnel: [w956] -> w951
                tunnel: [w955] -> w950
                tunnel: [w954] -> w949
                n288 = node-c288() -> ()  [unwired: 1 in, 1 out]
                n289 = case shown="True" "Read VC 840 1" {
                  tunnel: w958 -> [w962 w968]
                  tunnel: w957 -> [w963 w967]
                  tunnel: [w962 w966] -> w956
                  tunnel: [w963 w965] -> w955
                  tunnel: [0.0 ("Reading") w964] -> w954
                  frame False {
                    n290 = property on="Read VC 840 1" class="Bool (strict)"("Blinking"=FALSE) -> ()  [unwired: 2 in, 2 out]
                  }
                  frame True {
                    n291 = stacked-sequence {
                      tunnel: w968 -> [_ w975]
                      tunnel: w967 -> [_ w974]
                      tunnel: [_ w973] -> w966
                      tunnel: [_ w972] -> w965
                      tunnel: [_ w970] -> w964
                      frame #0 {
                        n292 = property on="Read VC 840 1" class="Bool (strict)"("Blinking"=TRUE) -> ()  [unwired: 2 in, 2 out]
                      }
                      frame #1 {
                        n293 = call "VC840_Read.vi"("error in (no error)"=w974, "VISA resource name"=w975) -> ("error out"=w972:errorcluster, "Unit"=→"Unit 1":string, "Reading"=w970:dbl, "VISA resource name out"=w973:refnum<visa-resource-name>, "Status"=→"Status 1":T4, "Mode"=→"Mode 1":enum16{"?", "Diode", "Beep", "DC", "AC"})  [unwired: 4 out]
                        "Reading 1" <- w970
                      }
                    }
                  }
                }
                n294 = node-c288() -> ()  [unwired: 1 in, 1 out]
              }
            }
            n295 = Tick Count (ms)() -> (millisecond timer value=w811:u32)
            n296 = Subtract(x=w811, y=w816) -> (x-y=w815:u32)
            n297 = Divide(x=w815, y=u32 1000) -> (x/y=w813:dbl)
            n298 = To Double Precision Float(number=w813) -> (double precision float=w817:dbl)
            "current time (s)" <- w817
            n299 = node-c288(w837) -> ()  [unwired: 1 out]
            n300 = node-c288(w852) -> ()  [unwired: 1 out]
            n301 = node-c288(w834) -> ()  [unwired: 1 out]
            n302 = node-c288(w848) -> ()  [unwired: 1 out]
          }
          frame #4 {
            n303 = Build Array (concatenate)(w1004, w1003) -> (w1002:dbl[])
            n304 = Greater?(x=w1003, y="Pressure Limit (mbar)") -> (0:w1007:bool)
            n305 = case shown="True" w1007 {
              frame False {
                n306 = property on="Standby" class="Bool (strict)"("DisabledEnum"=T8."Enabled" ("Disabled")) -> ()  [unwired: 2 in, 2 out]
              }
              frame True {
                n307 = property on="Standby" class="Bool (strict)"("Val(Sgnl)"=TRUE ("Standby"), "DisabledEnum"=T8."Disabled" ("Disabled")) -> ()  [unwired: 2 in, 2 out]
              }
            }
            n308 = call "Resistivity_Calculation.vi"("Reading 1 (V)"=w995, "Constant"="Constant", "Thickness (nm)"="Thickness (nm)", "Reading 2 (A)"=w1005) -> ("Resivtivity (Ohm*cm)"=w987:dbl, "Current"=w988:dbl, "Voltage"=w989:dbl)
            "Resistivity (Ohm*cm)" <- w987
            "Voltage (V)" <- w989
            "Current (A)" <- w988
            n309 = call "I3252_Edit_Temperature.vi"("Temp. String"=w1006) -> ("Temp. (°C)"=w998:dbl)
            "Temperature (°C)" <- w998
            n310 = Build Array (concatenate)(w1000, w1001) -> (w997:dbl[])
            n311 = Build Array (concatenate)(w999, w998) -> (w985:dbl[])
            n312 = Build Array (concatenate)(w996, w989) -> (w994:dbl[])
            n313 = Build Array (concatenate)(w993, w988) -> (w991:dbl[])
            n314 = Build Array (concatenate)(w992, w987) -> (w990:dbl[])
            n315 = Build Array(w989, w988, w987) -> (w986:dbl[])
          }
          frame #5 {
            n316 = Bundle(w1025, w1034) -> (→"Pressure":cluster{dbl[], dbl[]})  [unwired: 1 in]
            n317 = Bundle(w1025, w1024) -> (→"Temperature":cluster{dbl[], dbl[]})  [unwired: 1 in]
            n318 = Bundle(w1025, w1027) -> (→"Voltage":cluster{dbl[], dbl[]})  [unwired: 1 in]
            n319 = Bundle(w1025, w1028) -> (→"Current":cluster{dbl[], dbl[]})  [unwired: 1 in]
            n320 = Bundle(w1025, w1029) -> (→"Resistivity":cluster{dbl[], dbl[]})  [unwired: 1 in]
            n321 = Build Array (concatenate)(w1023, w1036, w1035, w1022) -> (w1044:dbl[])
            "appended array" <- w1044
          }
          frame #6 {
            n322 = case shown="True" "Write to File" {
              tunnel: [_ w1070] -> w1055
              tunnel: "File Path" -> [_ w1068]
              tunnel: w1047 -> [_ w1066]
              frame False {
                n323 = property on="Write to File" class="Bool (strict)"("Blinking"=FALSE) -> ()  [unwired: 2 in, 2 out]
              }
              frame True {
                n324 = flat-sequence {
                  tunnel: [w1072] -> w1069
                  tunnel: w1068 -> [w1072]
                  tunnel: [w1071] -> w1067
                  tunnel: w1066 -> [w1071]
                  tunnel: [w1077] -> w1070
                  tunnel: w1069 -> [w1076]
                  tunnel: w1067 -> [w1075]
                  frame #0 {
                    n325 = property on="Write to File" class="Bool (strict)"("Blinking"=TRUE) -> ()  [unwired: 2 in, 2 out]
                  }
                  frame #1 {
                    n326 = call-poly <vilib>:"Write To Spreadsheet File.vi"("format (%.3f)"="%g", "append to file? (new file:F)"=TRUE ("transpose? (no:F)"), "1D data"=w1075, "file path (dialog if empty)"=w1076) -> ("new file path (Not A Path if cancelled)"=w1077:path)  [unwired: 4 in]
                  }
                }
              }
            }
            n327 = Merge Errors(w1060, w1059, w1057) -> (w1058:errorcluster)
            n328 = call <vilib>:"Simple Error Handler.vi"("error in (no error)"=w1058) -> ("error?"=w1046:bool)  [unwired: 4 in, 4 out]
            n329 = local write "File Path"(w1055) -> ()
          }
          frame #7 {
            w1080 = u32 1000 ("y")
            n330 = Tick Count (ms)() -> (millisecond timer value=w1082:u32)
            n331 = Subtract(x=w1082, y=w1081) -> (x-y=w1083:u32)
            n332 = Divide(x=w1083, y=w1080) -> (x/y=→"loop time (s)":dbl)
            n333 = Subtract(x="Intervall (s)", y=u32 1) -> (x-y=w1084:u32)
            n334 = Multiply(x=w1084, y=w1080) -> (x*y=w1087:u32)
            n335 = Wait (ms)(milliseconds to wait=w1087) -> ()  [unwired: 1 out]
          }
          frame #8 {
            n336 = Tick Count (ms)() -> (millisecond timer value=w1104:u32)
            n337 = Subtract(x=w1104, y=w1102) -> (x-y=w1103:u32)
            n338 = Divide(x=w1103, y=w1101) -> (x/y=→"data logger intervall (s)":dbl)
          }
        }
      }
    }
    frame #4 {
      n339 = call "VC840_Close.vi"("error in (no error)"=w1121, "VISA resource name"=w1122) -> ("error out"=w1130:errorcluster)  [unwired: 9 in]
      n340 = call "VC840_Close.vi"("error in (no error)"=w1123, "VISA resource name"=w1124) -> ("error out"=w1128:errorcluster)  [unwired: 9 in]
      n341 = VISA Close(VISA resource name=w1126, error in (no error)=w1125) -> (error out=w1127:errorcluster)
      n342 = Merge Errors(w1127, w1128, w1130) -> (w1129:errorcluster)
      n343 = call <vilib>:"Simple Error Handler.vi"("error in (no error)"=w1129) -> ("error?"=w1119:bool)  [unwired: 1 in, 7 out]
      n344 = Stop(stop? (T)=w1119) -> ()
      "Error Out" <- w1120
    }
  }
